vi "BRig_RT_panel_manualTriggering_v0,90.vi"(0 "input_dataMTrig":u16[](array[numeric]), 6 "input_setValues":bool) -> (11 "output_Solenoid_R":bool, 13 "output_Solenoid_L":bool, 14 "output_dataMTrig":u16[](array[numeric]), 15 "output_Audio_L":bool, 16 "output_Audio_R":bool, 17 "output_CueLed":bool, 18 "output_Laser_l1":bool, 19 "output_Laser_l2":bool)   [LabVIEW 2014]
panel:
  in  "warmup_CueSwitch":bool
  out "SolenoidCal_I_R":bool
  out "SolenoidCal_I_L":bool
  in  "CueLed_T":u16=10 caption="Time [ms]"
  in  "Audio_T":u16=10 caption="Time [ms]"
  in  "count_warmup_R_reset":bool
  in  "count_warmup_L_reset":bool
  out "count_warmup_R":u16
  out "count_warmup_L":u16
  in  "warmup_struct":u8(slide) max=2 step=1 scale=0.0..2.0
  in  "warmup":bool caption="WarmUp"
  in  "CueLed":bool
  in  "Laser_Switch":bool
  in  "Laser_T":u16=10 caption="Time [ms]"
  in  "Laser":bool
  in  "Audio_R":bool caption="Trigger Audio"
  in  "Audio_L":bool caption="Trigger Audio"
  in  "RewCalib_R":bool caption="Calibrate_R"
  in  "RewCalib_L":bool caption="Calibrate_L"
  in  "Solenoid_T_R":u16=300 caption="Time [ms]"
  in  "Solenoid_T_L":u16=300 caption="Time [ms]"
  in  "Solenoid_R":bool caption="Solenoid"
  in  "Solenoid_L":bool caption="Solenoid"
  # "WarmUp"
  # "Cue then reward (no lick)\n \nLeft                    Right"
  # "Cue LED\n\nAudio"
  # "Manual Control"
  # "Solenoid\n \nLeft              Right"
  # "Speaker\n \nLeft                    Right"
  # "Laser 1  |  Laser 2"
  # "Cue LED"
  # "Time\n[ms]"
  # "Time\n[ms]"
  # "Power = Min"
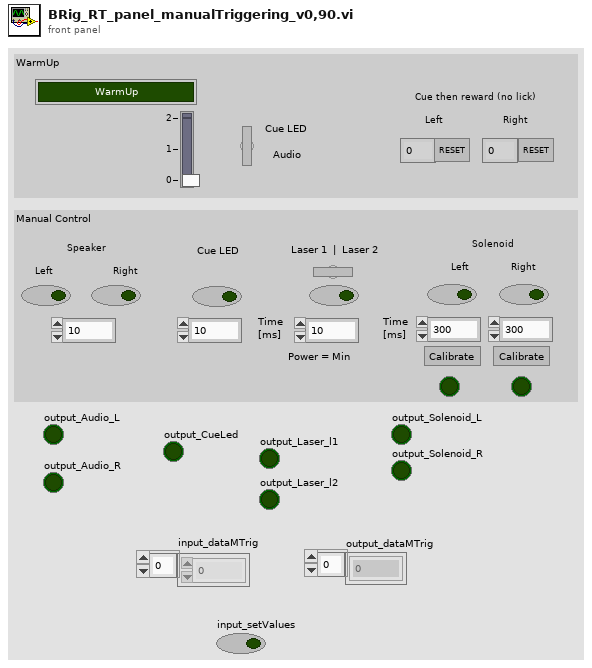
[diagram p1: front panel]
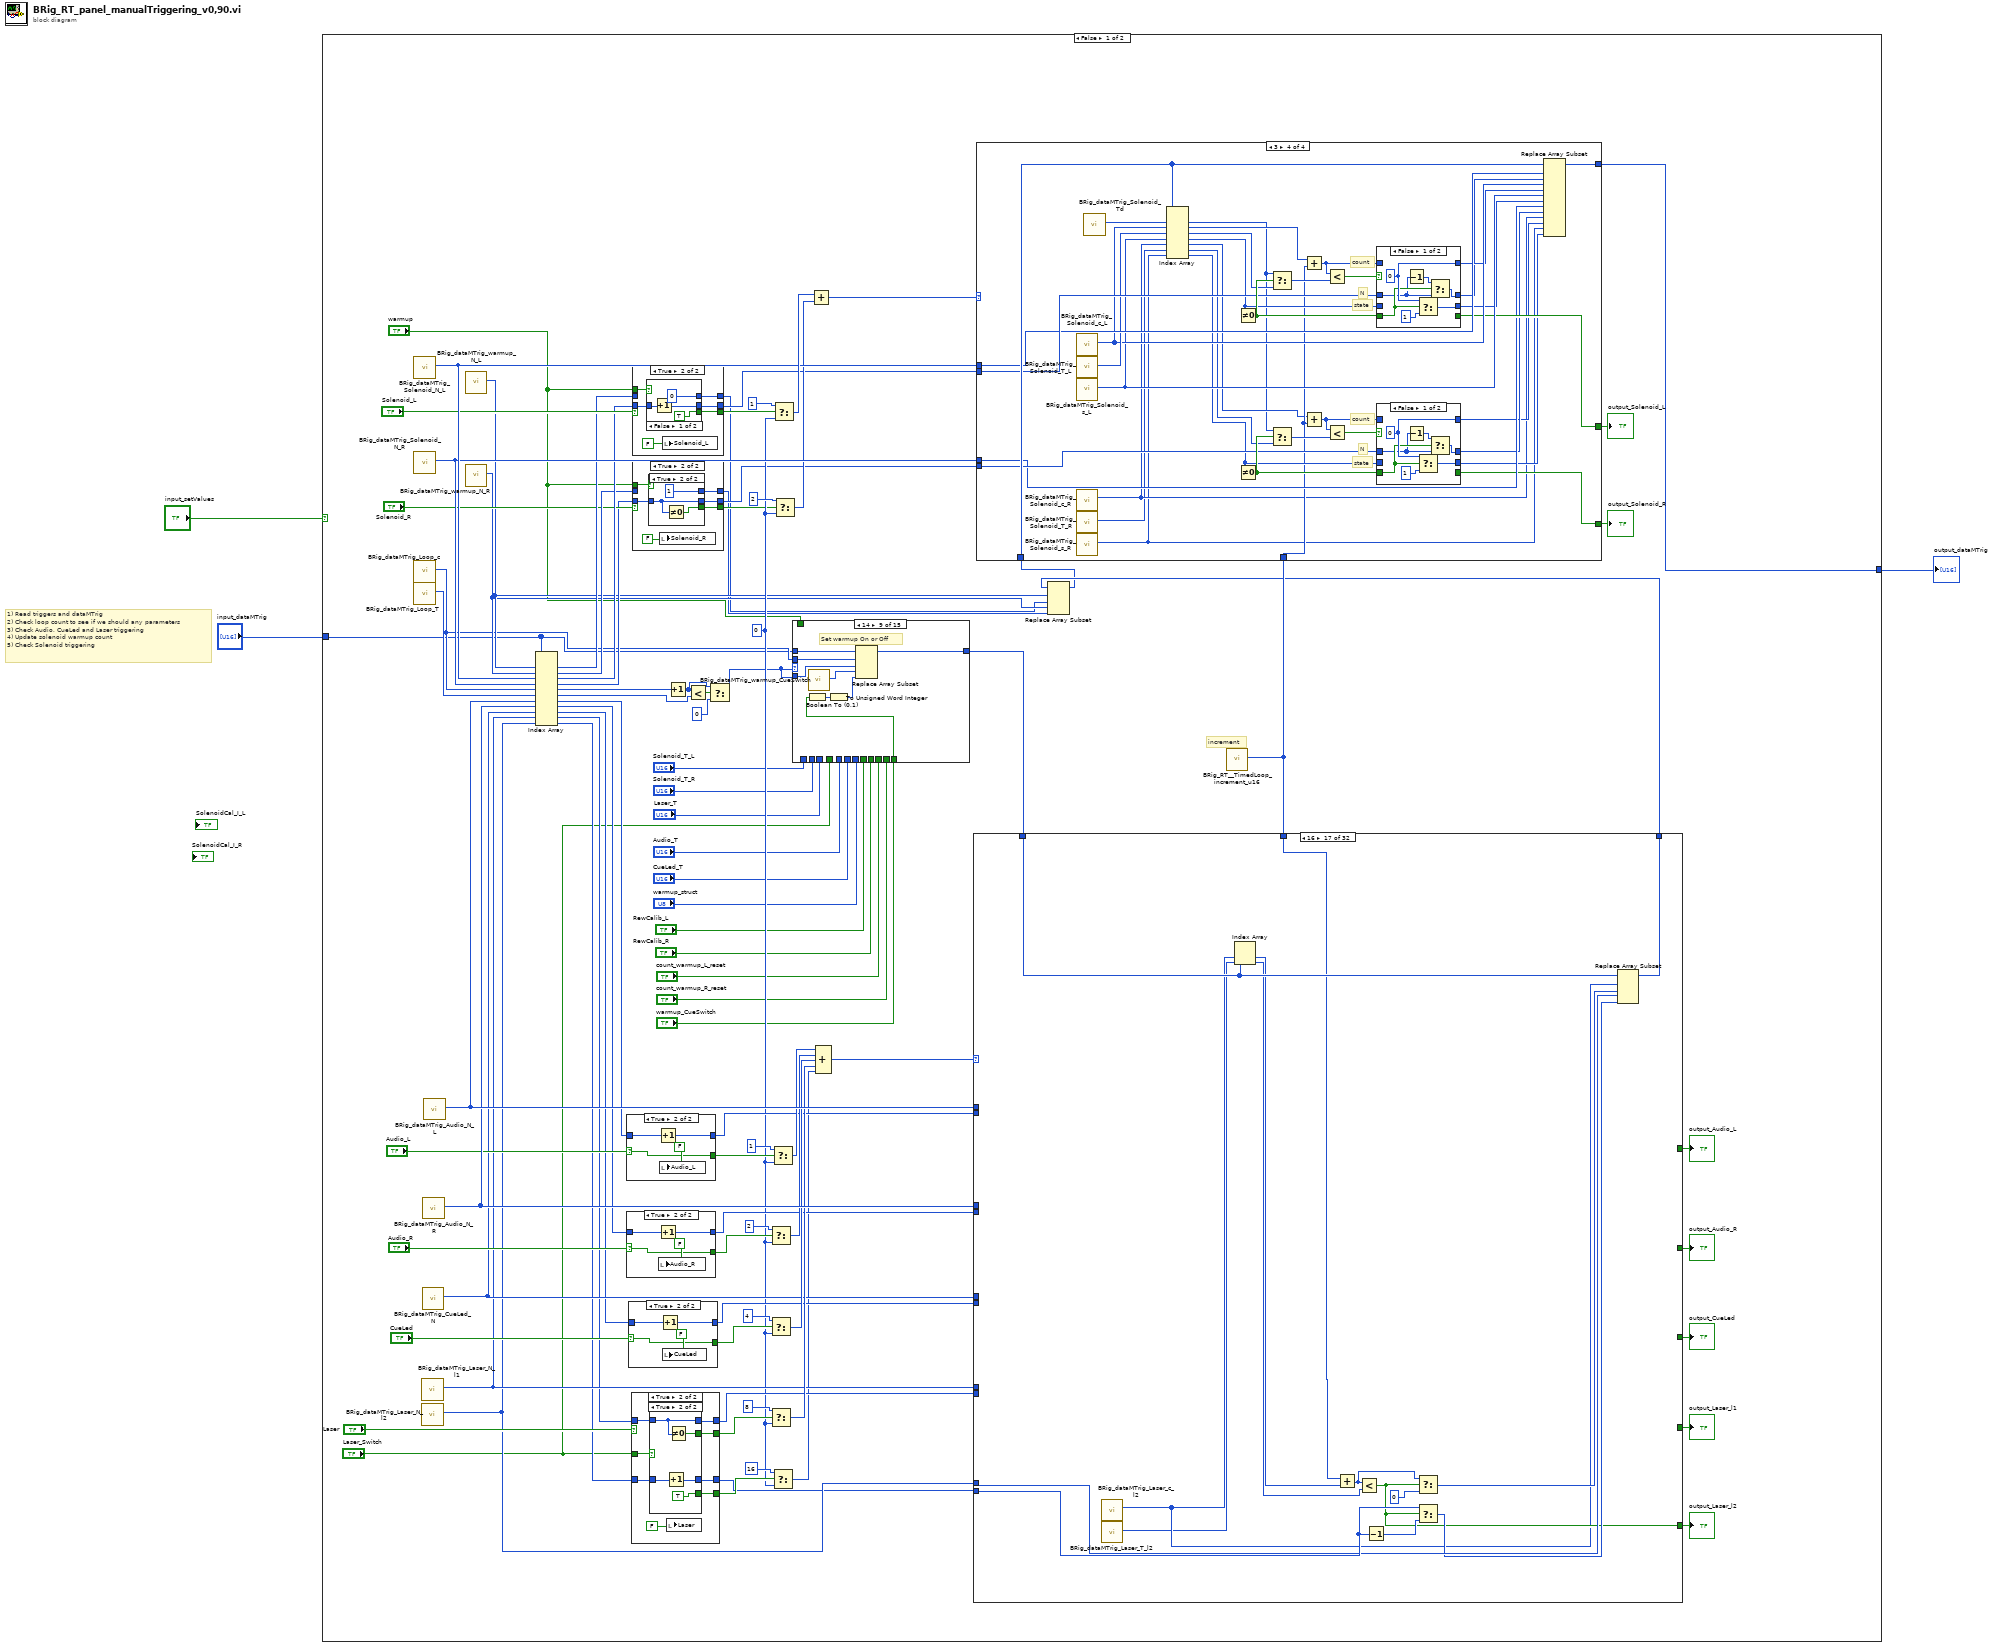
[diagram p0: block diagram]
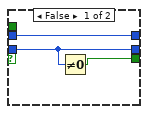
[diagram p2: hidden frame]
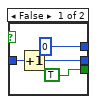
[diagram p3: hidden frame]
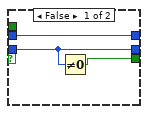
[diagram p4: hidden frame]
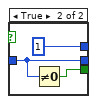
[diagram p5: hidden frame]
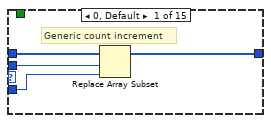
[diagram p6: hidden frame]
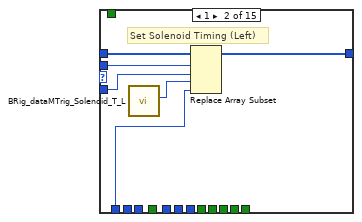
[diagram p7: hidden frame]
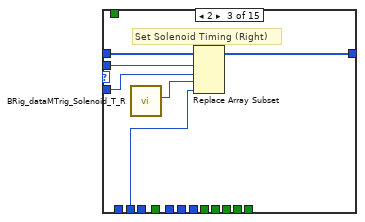
[diagram p8: hidden frame]
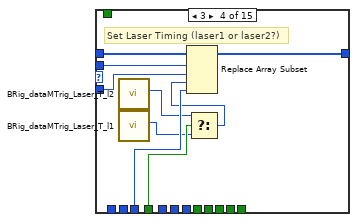
[diagram p9: hidden frame]
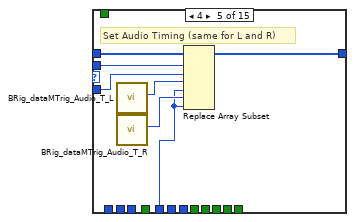
[diagram p10: hidden frame]
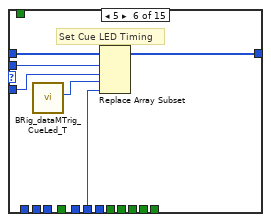
[diagram p11: hidden frame]
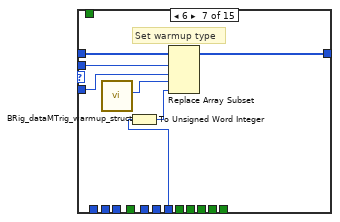
[diagram p12: hidden frame]
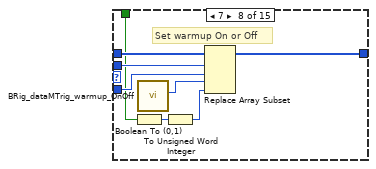
[diagram p13: hidden frame]
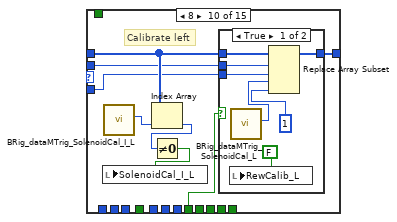
[diagram p14: hidden frame]
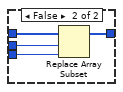
[diagram p15: hidden frame]
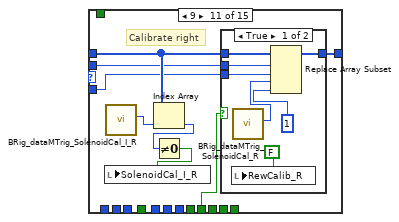
[diagram p16: hidden frame]
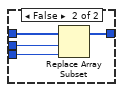
[diagram p17: hidden frame]
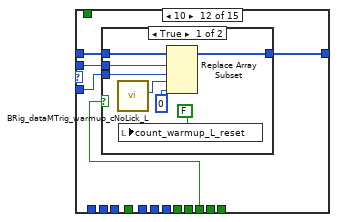
[diagram p18: hidden frame]
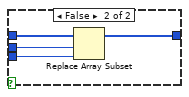
[diagram p19: hidden frame]
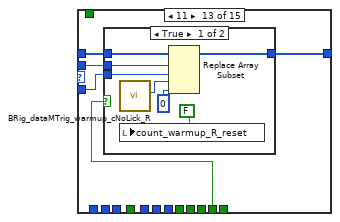
[diagram p20: hidden frame]
diagram:
  # "1) Read triggers and dataMTrig\n2) Check loop count to see if we should any parameters\n3) Check Audio, CueLed and Laser triggering\n4) Update solenoid warmup count\n5) Check Solenoid triggering"
  n1 = case shown="False" "input_setValues" {
    tunnel: [w54 w1492] -> w3
    tunnel: "input_dataMTrig" -> [w7 w1492]
    frame False {
      w39 = u8 0 ("f")
      # "increment"
      n2 = call "BRig_dataMTrig_Solenoid_N_L.vi"() -> ("output_Solenoid_N_L"=w48:i32)  [unwired: 11 in]
      n3 = call "BRig_dataMTrig_Solenoid_N_R.vi"() -> ("output_Solenoid_N_R"=w47:i32)  [unwired: 11 in]
      n4 = call "BRig_dataMTrig_Loop_c.vi"() -> ("output_Loop_c"=w9:i32)  [unwired: 11 in]
      n5 = call "BRig_dataMTrig_Loop_T.vi"() -> ("output_Loop_T"=w52:i32)  [unwired: 11 in]
      n6 = call "BRig_dataMTrig_Laser_N_l1.vi"() -> ("output_Laser_N_l1"=w73:i32)  [unwired: 11 in]
      n7 = call "BRig_dataMTrig_Laser_N_l2.vi"() -> ("output_Laser_N_l2"=w61:i32)  [unwired: 11 in]
      n8 = call "BRig_dataMTrig_CueLed_N.vi"() -> ("output_CueLed_N"=w74:i32)  [unwired: 11 in]
      n9 = call "BRig_dataMTrig_Audio_N_R.vi"() -> ("output_Audio_N_R"=w91:i32)  [unwired: 11 in]
      n10 = call "BRig_dataMTrig_Audio_N_L.vi"() -> ("output_Audio_N_L"=w92:i32)  [unwired: 11 in]
      n11 = call "BRig_dataMTrig_warmup_N_L.vi"() -> ("output_warmup_N_L"=w18:i32)  [unwired: 11 in]
      n12 = call "BRig_dataMTrig_warmup_N_R.vi"() -> ("output_warmup_N_R"=w17:i32)  [unwired: 11 in]
      n13 = Index Array(array=w7, index #1=w18, index #2=w17, index #3=w48, index #4=w47, index #5=w9, index #6=w52, index #7=w92, index #8=w91, index #9=w74, index #10=w73, index #11=w61) -> (element #1=w28:u16, element #2=w25:u16, element #3=w29:u16, element #4=w23:u16, element #5=w42:u16, element #6=w41:u16, element #7=w82:u16, element #8=w78:u16, element #9=w72:u16, element #10=w69:u16, element #11=w65:u16)
      n14 = case shown="True" "Audio_L" {
        selector: "Audio_L" -> [_ w434]
        tunnel: w82 -> [w433 w437]
        tunnel: [w433 w436] -> w81
        tunnel: [w432 w434] -> w80
        frame False {
          n15 = Not Equal To 0?(x=w433) -> (x != 0?=w432:bool)
        }
        frame True {
          n16 = Increment(x=w437) -> (x+1=w436:u16)
          n17 = local write "Audio_L"(FALSE) -> ()
        }
      }
      n18 = case shown="True" "Audio_R" {
        selector: "Audio_R" -> [_ w428]
        tunnel: w78 -> [w427 w431]
        tunnel: [w427 w430] -> w76
        tunnel: [w426 w428] -> w77
        frame False {
          n19 = Not Equal To 0?(x=w427) -> (x != 0?=w426:bool)
        }
        frame True {
          n20 = Increment(x=w431) -> (x+1=w430:u16)
          n21 = local write "Audio_R"(FALSE) -> ()
        }
      }
      n22 = case shown="True" "CueLed" {
        selector: "CueLed" -> [_ w422]
        tunnel: w72 -> [w421 w425]
        tunnel: [w421 w424] -> w71
        tunnel: [w420 w422] -> w70
        frame False {
          n23 = Not Equal To 0?(x=w421) -> (x != 0?=w420:bool)
        }
        frame True {
          n24 = Increment(x=w425) -> (x+1=w424:u16)
          n25 = local write "CueLed"(FALSE) -> ()
        }
      }
      n26 = case shown="True" "Laser" {
        tunnel: w69 -> [w401 w407]
        tunnel: [w401 w406] -> w67
        tunnel: [w400 w405] -> w66
        tunnel: w65 -> [w399 w404]
        tunnel: "Laser_Switch" -> [_ w408]
        tunnel: [w399 w402] -> w60
        tunnel: [w398 w403] -> w63
        frame False {
          n27 = Not Equal To 0?(x=w401) -> (x != 0?=w400:bool)
          n28 = Not Equal To 0?(x=w399) -> (x != 0?=w398:bool)
        }
        frame True {
          n29 = case shown="True" w408 {
            tunnel: w407 -> [w414 w419]
            tunnel: [w413 w419] -> w406
            tunnel: [TRUE w418] -> w405
            tunnel: [w411 w416] -> w402
            tunnel: w404 -> [w411 w417]
            tunnel: [w410 TRUE] -> w403
            frame False {
              n30 = Increment(x=w414) -> (x+1=w413:u16)
              n31 = Not Equal To 0?(x=w411) -> (x != 0?=w410:bool)
            }
            frame True {
              n32 = Increment(x=w417) -> (x+1=w416:u16)
              n33 = Not Equal To 0?(x=w419) -> (x != 0?=w418:bool)
            }
          }
          n34 = local write "Laser"(FALSE) -> ()
        }
      }
      n35 = case shown="True" "Solenoid_L" {
        tunnel: w29 -> [w113 w119]
        tunnel: [w113 w118] -> w26
        tunnel: [w112 w114] -> w27
        tunnel: "warmup" -> [_ w117]
        tunnel: [w111 w116] -> w15
        tunnel: w28 -> [w111 _]
        frame False {
          n36 = Not Equal To 0?(x=w113) -> (x != 0?=w112:bool)
        }
        frame True {
          n37 = case shown="False" w117 {
            tunnel: w119 -> [w123 w125]
            tunnel: [w122 w125] -> w118
            tunnel: [u16 0 u16 1] -> w116
            tunnel: [TRUE w124] -> w114
            frame False {
              n38 = Increment(x=w123) -> (x+1=w122:u16)
            }
            frame True {
              n39 = Not Equal To 0?(x=w125) -> (x != 0?=w124:bool)
            }
          }
          n40 = local write "Solenoid_L"(FALSE) -> ()
        }
      }
      n41 = case shown="True" "Solenoid_R" {
        tunnel: w23 -> [w97 w100]
        tunnel: [w97 w102] -> w21
        tunnel: [w96 w98] -> w22
        tunnel: "warmup" -> [_ w101]
        tunnel: [w95 w99] -> w16
        tunnel: w25 -> [w95 _]
        frame False {
          n42 = Not Equal To 0?(x=w97) -> (x != 0?=w96:bool)
        }
        frame True {
          n43 = case shown="True" w101 {
            tunnel: w100 -> [w107 w109]
            tunnel: [w106 w109] -> w102
            tunnel: [u16 0 u16 1] -> w99
            tunnel: [TRUE w108] -> w98
            frame False {
              n44 = Increment(x=w107) -> (x+1=w106:u16)
            }
            frame True {
              n45 = Not Equal To 0?(x=w109) -> (x != 0?=w108:bool)
            }
          }
          n46 = local write "Solenoid_R"(FALSE) -> ()
        }
      }
      n47 = Increment(x=w42) -> (x+1=w36:u16)
      n48 = Less?(x=w36, y=w41) -> (x < y?=w40:bool)
      n49 = Select(t=w36, s=w40, f=u16 0) -> (s? t:f=w31:u16)
      n50 = Select(t=u8 2, s=w77, f=w39) -> (s? t:f=w88:u8)
      n51 = Select(t=u8 4, s=w70, f=w39) -> (s? t:f=w87:u8)
      n52 = Select(t=u8 8, s=w66, f=w39) -> (s? t:f=w85:u8)
      n53 = Select(t=u8 1, s=w80, f=w39) -> (s? t:f=w89:u8)
      n54 = Select(t=u8 16, s=w63, f=w39) -> (s? t:f=w62:u8)
      n55 = Select(t=u8 1, s=w27, f=w39) -> (s? t:f=w50:u8)
      n56 = Select(t=u8 2, s=w22, f=w39) -> (s? t:f=w45:u8)
      n57 = case shown="14" w31 {
        tunnel: w7 -> [w130 w136 w142 w151 w158 w164 w171 w179 w187 w192 w211 w230 w246 w260 w266]
        tunnel: [w129 w135 w141 w150 w157 w163 w170 w178 w186 w190 w210 w229 w245 w263 w269] -> w37
        tunnel: w31 -> [w127 w133 w139 w148 w155 w161 w168 w176 w184 w188 w208 w227 w243 w261 w267]
        tunnel: w9 -> [w128 w134 w140 w149 w156 w162 w169 w177 w185 w189 w209 w228 w244 w262 w268]
        tunnel: "Solenoid_T_L" -> [_ w131 _ _ _ _ _ _ _ _ _ _ _ _ _]
        tunnel: "Solenoid_T_R" -> [_ _ w137 _ _ _ _ _ _ _ _ _ _ _ _]
        tunnel: "Laser_T" -> [_ _ _ w147 _ _ _ _ _ _ _ _ _ _ _]
        tunnel: "Laser_Switch" -> [_ _ _ w146 _ _ _ _ _ _ _ _ _ _ _]
        tunnel: "Audio_T" -> [_ _ _ _ w152 _ _ _ _ _ _ _ _ _ _]
        tunnel: "CueLed_T" -> [_ _ _ _ _ w159 _ _ _ _ _ _ _ _ _]
        tunnel: "warmup_struct" -> [_ _ _ _ _ _ w166 _ _ _ _ _ _ _ _]
        tunnel: "warmup" -> [_ _ _ _ _ _ _ w172 _ _ _ _ _ _ _]
        tunnel: "RewCalib_L" -> [_ _ _ _ _ _ _ _ _ w191 _ _ _ _ _]
        tunnel: "RewCalib_R" -> [_ _ _ _ _ _ _ _ _ _ w207 _ _ _ _]
        tunnel: "count_warmup_L_reset" -> [_ _ _ _ _ _ _ _ _ _ _ w226 _ _ _]
        tunnel: "count_warmup_R_reset" -> [_ _ _ _ _ _ _ _ _ _ _ _ w242 _ _]
        tunnel: "warmup_CueSwitch" -> [_ _ _ _ _ _ _ _ w181 _ _ _ _ _ _]
        frame 0, Default {
          # "Generic count increment"
          n58 = Replace Array Subset(array=w130, new element=w127, index=w128) -> (w129:u16[])
        }
        frame 1 {
          # "Set Solenoid Timing (Left)"
          n59 = call "BRig_dataMTrig_Solenoid_T_L.vi"() -> ("output_Solenoid_T_L"=w132:i32)  [unwired: 11 in]
          n60 = Replace Array Subset(array=w136, new element #1=w133, index #1=w134, new element #2=w131, index #2=w132) -> (w135:u16[])
        }
        frame 2 {
          # "Set Solenoid Timing (Right)"
          n61 = call "BRig_dataMTrig_Solenoid_T_R.vi"() -> ("output_Solenoid_T_R"=w138:i32)  [unwired: 11 in]
          n62 = Replace Array Subset(array=w142, new element #1=w139, index #1=w140, new element #2=w137, index #2=w138) -> (w141:u16[])
        }
        frame 3 {
          # "Set Laser Timing (laser1 or laser2?)"
          n63 = call "BRig_dataMTrig_Laser_T_l2.vi"() -> ("output_Laser_T_l2"=w144:i32)  [unwired: 11 in]
          n64 = call "BRig_dataMTrig_Laser_T_l1.vi"() -> ("output_Laser_T_l1"=w145:i32)  [unwired: 11 in]
          n65 = Select(t=w144, s=w146, f=w145) -> (s? t:f=w143:i32)
          n66 = Replace Array Subset(array=w151, new element #1=w148, index #1=w149, new element #2=w147, index #2=w143) -> (w150:u16[])
        }
        frame 4 {
          # "Set Audio Timing (same for L and R)"
          n67 = call "BRig_dataMTrig_Audio_T_L.vi"() -> ("output_Audio_T_L"=w154:i32)  [unwired: 11 in]
          n68 = call "BRig_dataMTrig_Audio_T_R.vi"() -> ("output_Audio_T_R"=w153:i32)  [unwired: 11 in]
          n69 = Replace Array Subset(array=w158, new element #1=w155, index #1=w156, new element #2=w152, index #2=w154, new element #3=w152, index #3=w153) -> (w157:u16[])
        }
        frame 5 {
          # "Set Cue LED Timing"
          n70 = call "BRig_dataMTrig_CueLed_T.vi"() -> ("output_CueLed_T"=w160:i32)  [unwired: 11 in]
          n71 = Replace Array Subset(array=w164, new element #1=w161, index #1=w162, new element #2=w159, index #2=w160) -> (w163:u16[])
        }
        frame 6 {
          # "Set warmup type"
          n72 = call "BRig_dataMTrig_warmup_struct.vi"() -> ("output_warmup_struct"=w167:i32)  [unwired: 11 in]
          n73 = To Unsigned Word Integer(number=w166) -> (unsigned 16bit integer=w165:u16)
          n74 = Replace Array Subset(array=w171, new element #1=w168, index #1=w169, new element #2=w165, index #2=w167) -> (w170:u16[])
        }
        frame 7 {
          # "Set warmup On or Off"
          n75 = Boolean To (0,1)(Boolean=w172) -> (0, 1=w173:i16)
          n76 = call "BRig_dataMTrig_warmup_OnOff.vi"() -> ("output_warmup_OnOff"=w174:i32)  [unwired: 11 in]
          n77 = To Unsigned Word Integer(number=w173) -> (unsigned 16bit integer=w175:u16)
          n78 = Replace Array Subset(array=w179, new element #1=w176, index #1=w177, new element #2=w175, index #2=w174) -> (w178:u16[])
        }
        frame 14 {
          # "Set warmup On or Off"
          n79 = Boolean To (0,1)(Boolean=w181) -> (0, 1=w182:i16)
          n80 = call "BRig_dataMTrig_warmup_CueSwitch.vi"() -> ("output_warmup_CueSwitch"=w180:i32)  [unwired: 11 in]
          n81 = To Unsigned Word Integer(number=w182) -> (unsigned 16bit integer=w183:u16)
          n82 = Replace Array Subset(array=w187, new element #1=w184, index #1=w185, new element #2=w183, index #2=w180) -> (w186:u16[])
        }
        frame 8 {
          # "Calibrate left"
          n83 = call "BRig_dataMTrig_SolenoidCal_I_L.vi"() -> ("output_SolenoidCal_I_L"=w195:i32)  [unwired: 11 in]
          n84 = Index Array(array=w192, index=w195) -> (element=w194:u16)
          n85 = Not Equal To 0?(x=w194) -> (x != 0?=w193:bool)
          n86 = local write "SolenoidCal_I_L"(w193) -> ()
          n87 = case shown="True" w191 {
            tunnel: w192 -> [w201 w206]
            tunnel: [w200 w205] -> w190
            tunnel: w189 -> [w199 w204]
            tunnel: w188 -> [w198 w203]
            frame True {
              n88 = local write "RewCalib_L"(FALSE) -> ()
              n89 = call "BRig_dataMTrig_SolenoidCal_L.vi"() -> ("output_SolenoidCal_L"=w197:i32)  [unwired: 11 in]
              n90 = Replace Array Subset(array=w201, new element #1=w198, index #1=w199, new element #2=u16 1 ("new element/subarray"), index #2=w197) -> (w200:u16[])
            }
            frame False {
              n91 = Replace Array Subset(array=w206, new element=w203, index=w204) -> (w205:u16[])
            }
          }
        }
        frame 9 {
          # "Calibrate right"
          n92 = call "BRig_dataMTrig_SolenoidCal_I_R.vi"() -> ("output_SolenoidCal_I_R"=w214:i32)  [unwired: 11 in]
          n93 = Index Array(array=w211, index=w214) -> (element=w213:u16)
          n94 = Not Equal To 0?(x=w213) -> (x != 0?=w212:bool)
          n95 = local write "SolenoidCal_I_R"(w212) -> ()
          n96 = case shown="True" w207 {
            tunnel: w211 -> [w220 w225]
            tunnel: [w219 w224] -> w210
            tunnel: w209 -> [w218 w223]
            tunnel: w208 -> [w217 w222]
            frame True {
              n97 = local write "RewCalib_R"(FALSE) -> ()
              n98 = call "BRig_dataMTrig_SolenoidCal_R.vi"() -> ("output_SolenoidCal_R"=w216:i32)  [unwired: 11 in]
              n99 = Replace Array Subset(array=w220, new element #1=w217, index #1=w218, new element #2=u16 1 ("new element/subarray"), index #2=w216) -> (w219:u16[])
            }
            frame False {
              n100 = Replace Array Subset(array=w225, new element=w222, index=w223) -> (w224:u16[])
            }
          }
        }
        frame 10 {
          n101 = case shown="True" w226 {
            tunnel: w230 -> [w237 w241]
            tunnel: [w236 w240] -> w229
            tunnel: w228 -> [w235 w239]
            tunnel: w227 -> [w234 w238]
            frame True {
              n102 = call "BRig_dataMTrig_warmup_cNoLick_L.vi"() -> ("output_warmup_cNoLick_L"=w233:i32)  [unwired: 11 in]
              n103 = local write "count_warmup_L_reset"(FALSE ("count_warmup_L_reset")) -> ()
              n104 = Replace Array Subset(array=w237, new element #1=w234, index #1=w235, new element #2=u16 0 ("new element/subarray"), index #2=w233) -> (w236:u16[])
            }
            frame False {
              n105 = Replace Array Subset(array=w241, new element=w238, index=w239) -> (w240:u16[])
            }
          }
        }
        frame 11 {
          n106 = case shown="True" w242 {
            tunnel: w246 -> [w253 w257]
            tunnel: [w252 w256] -> w245
            tunnel: w244 -> [w251 w255]
            tunnel: w243 -> [w250 w254]
            frame True {
              n107 = call "BRig_dataMTrig_warmup_cNoLick_R.vi"() -> ("output_warmup_cNoLick_R"=w247:i32)  [unwired: 11 in]
              n108 = local write "count_warmup_R_reset"(FALSE ("count_warmup_L_reset")) -> ()
              n109 = Replace Array Subset(array=w253, new element #1=w250, index #1=w251, new element #2=u16 0 ("new element/subarray"), index #2=w247) -> (w252:u16[])
            }
            frame False {
              n110 = Replace Array Subset(array=w257, new element=w254, index=w255) -> (w256:u16[])
            }
          }
        }
        frame 12 {
          n111 = call "BRig_dataMTrig_warmup_cNoLick_L.vi"() -> ("output_warmup_cNoLick_L"=w259:i32)  [unwired: 11 in]
          n112 = Replace Array Subset(array=w260, new element=w261, index=w262) -> (w263:u16[])
          n113 = Index Array(array=w260, index=w259) -> (element=→"count_warmup_L":u16)
        }
        frame 13 {
          n114 = call "BRig_dataMTrig_warmup_cNoLick_R.vi"() -> ("output_warmup_cNoLick_R"=w265:i32)  [unwired: 11 in]
          n115 = Replace Array Subset(array=w266, new element=w267, index=w268) -> (w269:u16[])
          n116 = Index Array(array=w266, index=w265) -> (element=→"count_warmup_R":u16)
        }
      }
      n117 = Add(x=w50, y=w45) -> (x+y=w49:u8)
      n118 = Compound Arithmetic op=ADD(w89, w88, w87, w85, w62) -> (w84:u8)
      n119 = call "BRig_RT__TimedLoop_increment_u16.vi"() -> ("output_increment__u16"=w53:u16)  [unwired: 11 in]
      n120 = case shown="16" w84 {
        tunnel: w37 -> [w438 w443 w458 w476 w502 w524 w547 w577 w618 w636 w669 w693 w731 w767 w800 w842 w882 w900 w927 w957 w995 w1029 w1064 w1106 w1158 w1194 w1233 w1281 w1319 w1367 w1412 w1466]
        tunnel: w53 -> [_ w444 w459 w477 w503 w525 w548 w578 w606 w626 w655 w680 w716 w750 w782 w821 w874 w891 w918 w945 w984 w1018 w1050 w1089 w1138 w1172 w1211 w1257 w1294 w1340 w1384 w1435]
        tunnel: [w438 w442 w457 w475 w501 w523 w546 w576 w617 w635 w668 w692 w730 w766 w799 w841 w881 w899 w926 w956 w994 w1028 w1063 w1105 w1157 w1193 w1232 w1280 w1318 w1366 w1411 w1465] -> w20
        tunnel: w92 -> [_ w440 _ w472 _ w520 _ w572 _ w633 _ w689 _ w744 _ w837 _ w897 _ w953 _ w1025 _ w1101 _ w1162 _ w1241 _ w1331 _ w1461]
        tunnel: w81 -> [_ w439 _ w471 _ w519 _ w571 _ w632 _ w688 _ w763 _ w836 _ w896 _ w952 _ w1024 _ w1100 _ w1191 _ w1277 _ w1363 _ w1460]
        tunnel: [_ w441 _ w474 _ w522 _ w575 _ w634 _ w691 _ w765 _ w840 _ w898 _ w955 _ w1027 _ w1104 _ w1192 _ w1279 _ w1365 _ w1464] -> w59
        tunnel: [_ _ w456 w473 _ _ w545 w574 _ _ w667 w690 _ _ w798 w839 _ _ w925 w954 _ _ w1062 w1103 _ _ w1231 w1278 _ _ w1410 w1463] -> w58
        tunnel: [_ _ _ _ w500 w521 w544 w573 _ _ _ _ w729 w764 w797 w838 _ _ _ _ w993 w1026 w1061 w1102 _ _ _ _ w1317 w1364 w1409 w1462] -> w57
        tunnel: w91 -> [_ _ w455 w470 _ _ w543 w570 _ _ w649 w687 _ _ w796 w835 _ _ w924 w951 _ _ w1060 w1099 _ _ w1202 w1245 _ _ w1408 w1459]
        tunnel: w76 -> [_ _ w454 w469 _ _ w542 w569 _ _ w666 w686 _ _ w795 w834 _ _ w923 w950 _ _ w1059 w1098 _ _ w1230 w1276 _ _ w1407 w1458]
        tunnel: w74 -> [_ _ _ _ w499 w514 w541 w568 _ _ _ _ w728 w762 w794 w833 _ _ _ _ w992 w1015 w1058 w1097 _ _ _ _ w1316 w1362 w1406 w1457]
        tunnel: w71 -> [_ _ _ _ w498 w518 w540 w567 _ _ _ _ w727 w761 w793 w832 _ _ _ _ w991 w1023 w1057 w1096 _ _ _ _ w1315 w1361 w1405 w1456]
        tunnel: w73 -> [_ _ _ _ _ _ _ _ w611 w622 w660 w676 w721 w755 w787 w826 _ _ _ _ _ _ _ _ w1151 w1185 w1224 w1270 w1309 w1355 w1399 w1450]
        tunnel: w67 -> [_ _ _ _ _ _ _ _ w613 w628 w662 w682 w723 w757 w789 w828 _ _ _ _ _ _ _ _ w1153 w1187 w1226 w1272 w1311 w1357 w1401 w1452]
        tunnel: [_ _ _ _ _ _ _ _ w612 w627 w661 w681 w722 w756 w788 w827 _ _ _ _ _ _ _ _ w1152 w1186 w1225 w1271 w1310 w1356 w1400 w1451] -> w56
        tunnel: w61 -> [_ _ _ _ _ _ _ _ _ _ _ _ _ _ _ _ w872 w888 w915 w940 w979 w1012 w1047 w1086 w1136 w1170 w1209 w1255 w1292 w1338 w1382 w1433]
        tunnel: w60 -> [_ _ _ _ _ _ _ _ _ _ _ _ _ _ _ _ w877 w892 w919 w946 w985 w1019 w1051 w1090 w1141 w1175 w1214 w1260 w1297 w1343 w1387 w1438]
        tunnel: [_ _ _ _ _ _ _ _ _ _ _ _ _ _ _ _ w870 w890 w917 w944 w983 w1017 w1049 w1088 w1134 w1168 w1207 w1253 w1290 w1336 w1380 w1431] -> w55
        frame 0, Default {
        }
        frame 1 {
          # "Audio_L"
          # "Tcycle"
          # "count"
          n121 = call "BRig_dataMTrig_Audio_c_L.vi"() -> ("output_Audio_c_L"=w445:i32)  [unwired: 11 in]
          n122 = call "BRig_dataMTrig_Audio_T_L.vi"() -> ("output_Audio_T_L"=w450:i32)  [unwired: 11 in]
          n123 = Index Array(array=w443, index #1=w445, index #2=w450) -> (element #1=w449:u16, element #2=w448:u16)
          n124 = Add(x=w444, y=w449) -> (x+y=w452:u16)
          n125 = Less?(x=w452, y=w448) -> (x < y?=w441:bool)
          n126 = Decrement(x=w439) -> (x-1=w453:u16)
          n127 = Select(t=w452, s=w441, f=u16 0) -> (s? t:f=w447:u16)
          n128 = Select(t=w439, s=w441, f=w453) -> (s? t:f=w446:u16)
          n129 = Replace Array Subset(array=w443, new element #1=w447, index #1=w445, new element #2=w446, index #2=w440) -> (w442:u16[])
        }
        frame 2 {
          # "Audio_R"
          # "Tcycle"
          # "count"
          n130 = call "BRig_dataMTrig_Audio_c_R.vi"() -> ("output_Audio_c_R"=w462:i32)  [unwired: 11 in]
          n131 = call "BRig_dataMTrig_Audio_T_R.vi"() -> ("output_Audio_T_R"=w463:i32)  [unwired: 11 in]
          n132 = Index Array(array=w458, index #1=w462, index #2=w463) -> (element #1=w465:u16, element #2=w464:u16)
          n133 = Add(x=w459, y=w465) -> (x+y=w467:u16)
          n134 = Less?(x=w467, y=w464) -> (x < y?=w456:bool)
          n135 = Decrement(x=w454) -> (x-1=w468:u16)
          n136 = Select(t=w467, s=w456, f=u16 0) -> (s? t:f=w461:u16)
          n137 = Select(t=w454, s=w456, f=w468) -> (s? t:f=w460:u16)
          n138 = Replace Array Subset(array=w458, new element #1=w461, index #1=w462, new element #2=w460, index #2=w455) -> (w457:u16[])
        }
        frame 3 {
          # "Audio_R"
          # "Tcycle"
          # "count"
          # "Audio_L"
          # "Tcycle"
          # "count"
          n139 = call "BRig_dataMTrig_Audio_c_L.vi"() -> ("output_Audio_c_L"=w487:i32)  [unwired: 11 in]
          n140 = call "BRig_dataMTrig_Audio_T_L.vi"() -> ("output_Audio_T_L"=w492:i32)  [unwired: 11 in]
          n141 = call "BRig_dataMTrig_Audio_c_R.vi"() -> ("output_Audio_c_R"=w480:i32)  [unwired: 11 in]
          n142 = call "BRig_dataMTrig_Audio_T_R.vi"() -> ("output_Audio_T_R"=w481:i32)  [unwired: 11 in]
          n143 = Index Array(array=w476, index #1=w487, index #2=w492, index #3=w480, index #4=w481) -> (element #1=w491:u16, element #2=w490:u16, element #3=w483:u16, element #4=w482:u16)
          n144 = Add(x=w477, y=w491) -> (x+y=w494:u16)
          n145 = Add(x=w477, y=w483) -> (x+y=w485:u16)
          n146 = Less?(x=w494, y=w490) -> (x < y?=w474:bool)
          n147 = Less?(x=w485, y=w482) -> (x < y?=w473:bool)
          n148 = Decrement(x=w471) -> (x-1=w495:u16)
          n149 = Decrement(x=w469) -> (x-1=w486:u16)
          n150 = Select(t=w494, s=w474, f=u16 0) -> (s? t:f=w489:u16)
          n151 = Select(t=w471, s=w474, f=w495) -> (s? t:f=w488:u16)
          n152 = Select(t=w485, s=w473, f=u16 0) -> (s? t:f=w479:u16)
          n153 = Select(t=w469, s=w473, f=w486) -> (s? t:f=w478:u16)
          n154 = Replace Array Subset(array=w476, new element #1=w489, index #1=w487, new element #2=w488, index #2=w472, new element #3=w479, index #3=w480, new element #4=w478, index #4=w470) -> (w475:u16[])
        }
        frame 4 {
          n155 = call "BRig_dataMTrig_CueLed_c.vi"() -> ("output_CueLed_c"=w497:i32)  [unwired: 11 in]
          n156 = call "BRig_dataMTrig_CueLed_T.vi"() -> ("output_CueLed_T"=w496:i32)  [unwired: 11 in]
          n157 = Index Array(array=w502, index #1=w497, index #2=w496) -> (element #1=w507:u16, element #2=w506:u16)
          n158 = Add(x=w503, y=w507) -> (x+y=w509:u16)
          n159 = Less?(x=w509, y=w506) -> (x < y?=w500:bool)
          n160 = Decrement(x=w498) -> (x-1=w510:u16)
          n161 = Select(t=w509, s=w500, f=u16 0) -> (s? t:f=w505:u16)
          n162 = Select(t=w498, s=w500, f=w510) -> (s? t:f=w504:u16)
          n163 = Replace Array Subset(array=w502, new element #1=w505, index #1=w497, new element #2=w504, index #2=w499) -> (w501:u16[])
        }
        frame 5 {
          # "Audio_L"
          # "Tcycle"
          # "count"
          n164 = call "BRig_dataMTrig_CueLed_c.vi"() -> ("output_CueLed_c"=w512:i32)  [unwired: 11 in]
          n165 = call "BRig_dataMTrig_CueLed_T.vi"() -> ("output_CueLed_T"=w511:i32)  [unwired: 11 in]
          n166 = call "BRig_dataMTrig_Audio_c_L.vi"() -> ("output_Audio_c_L"=w529:i32)  [unwired: 11 in]
          n167 = call "BRig_dataMTrig_Audio_T_L.vi"() -> ("output_Audio_T_L"=w534:i32)  [unwired: 11 in]
          n168 = Index Array(array=w524, index #1=w529, index #2=w534, index #3=w512, index #4=w511) -> (element #1=w533:u16, element #2=w532:u16, element #3=w517:u16, element #4=w516:u16)
          n169 = Add(x=w525, y=w533) -> (x+y=w536:u16)
          n170 = Add(x=w525, y=w517) -> (x+y=w527:u16)
          n171 = Less?(x=w536, y=w532) -> (x < y?=w522:bool)
          n172 = Less?(x=w527, y=w516) -> (x < y?=w521:bool)
          n173 = Decrement(x=w519) -> (x-1=w537:u16)
          n174 = Decrement(x=w518) -> (x-1=w528:u16)
          n175 = Select(t=w536, s=w522, f=u16 0) -> (s? t:f=w531:u16)
          n176 = Select(t=w519, s=w522, f=w537) -> (s? t:f=w530:u16)
          n177 = Select(t=w527, s=w521, f=u16 0) -> (s? t:f=w515:u16)
          n178 = Select(t=w518, s=w521, f=w528) -> (s? t:f=w513:u16)
          n179 = Replace Array Subset(array=w524, new element #1=w531, index #1=w529, new element #2=w530, index #2=w520, new element #3=w515, index #3=w512, new element #4=w513, index #4=w514) -> (w523:u16[])
        }
        frame 6 {
          # "Audio_R"
          # "Tcycle"
          # "count"
          n180 = call "BRig_dataMTrig_CueLed_c.vi"() -> ("output_CueLed_c"=w539:i32)  [unwired: 11 in]
          n181 = call "BRig_dataMTrig_CueLed_T.vi"() -> ("output_CueLed_T"=w538:i32)  [unwired: 11 in]
          n182 = call "BRig_dataMTrig_Audio_c_R.vi"() -> ("output_Audio_c_R"=w558:i32)  [unwired: 11 in]
          n183 = call "BRig_dataMTrig_Audio_T_R.vi"() -> ("output_Audio_T_R"=w559:i32)  [unwired: 11 in]
          n184 = Index Array(array=w547, index #1=w558, index #2=w559, index #3=w539, index #4=w538) -> (element #1=w561:u16, element #2=w560:u16, element #3=w552:u16, element #4=w551:u16)
          n185 = Add(x=w548, y=w561) -> (x+y=w563:u16)
          n186 = Add(x=w548, y=w552) -> (x+y=w554:u16)
          n187 = Less?(x=w563, y=w560) -> (x < y?=w545:bool)
          n188 = Less?(x=w554, y=w551) -> (x < y?=w544:bool)
          n189 = Decrement(x=w542) -> (x-1=w564:u16)
          n190 = Decrement(x=w540) -> (x-1=w555:u16)
          n191 = Select(t=w563, s=w545, f=u16 0) -> (s? t:f=w557:u16)
          n192 = Select(t=w542, s=w545, f=w564) -> (s? t:f=w556:u16)
          n193 = Select(t=w554, s=w544, f=u16 0) -> (s? t:f=w550:u16)
          n194 = Select(t=w540, s=w544, f=w555) -> (s? t:f=w549:u16)
          n195 = Replace Array Subset(array=w547, new element #1=w557, index #1=w558, new element #2=w556, index #2=w543, new element #3=w550, index #3=w539, new element #4=w549, index #4=w541) -> (w546:u16[])
        }
        frame 7 {
          # "Audio_R"
          # "Tcycle"
          # "count"
          # "Audio_L"
          # "Tcycle"
          # "count"
          n196 = call "BRig_dataMTrig_CueLed_c.vi"() -> ("output_CueLed_c"=w566:i32)  [unwired: 11 in]
          n197 = call "BRig_dataMTrig_CueLed_T.vi"() -> ("output_CueLed_T"=w565:i32)  [unwired: 11 in]
          n198 = call "BRig_dataMTrig_Audio_c_L.vi"() -> ("output_Audio_c_L"=w595:i32)  [unwired: 11 in]
          n199 = call "BRig_dataMTrig_Audio_T_L.vi"() -> ("output_Audio_T_L"=w600:i32)  [unwired: 11 in]
          n200 = call "BRig_dataMTrig_Audio_c_R.vi"() -> ("output_Audio_c_R"=w588:i32)  [unwired: 11 in]
          n201 = call "BRig_dataMTrig_Audio_T_R.vi"() -> ("output_Audio_T_R"=w589:i32)  [unwired: 11 in]
          n202 = Index Array(array=w577, index #1=w595, index #2=w600, index #3=w588, index #4=w589, index #5=w566, index #6=w565) -> (element #1=w599:u16, element #2=w598:u16, element #3=w591:u16, element #4=w590:u16, element #5=w582:u16, element #6=w581:u16)
          n203 = Add(x=w578, y=w599) -> (x+y=w602:u16)
          n204 = Add(x=w578, y=w591) -> (x+y=w593:u16)
          n205 = Add(x=w578, y=w582) -> (x+y=w584:u16)
          n206 = Less?(x=w602, y=w598) -> (x < y?=w575:bool)
          n207 = Less?(x=w593, y=w590) -> (x < y?=w574:bool)
          n208 = Less?(x=w584, y=w581) -> (x < y?=w573:bool)
          n209 = Decrement(x=w571) -> (x-1=w603:u16)
          n210 = Decrement(x=w569) -> (x-1=w594:u16)
          n211 = Decrement(x=w567) -> (x-1=w585:u16)
          n212 = Select(t=w602, s=w575, f=u16 0) -> (s? t:f=w597:u16)
          n213 = Select(t=w571, s=w575, f=w603) -> (s? t:f=w596:u16)
          n214 = Select(t=w593, s=w574, f=u16 0) -> (s? t:f=w587:u16)
          n215 = Select(t=w569, s=w574, f=w594) -> (s? t:f=w586:u16)
          n216 = Select(t=w584, s=w573, f=u16 0) -> (s? t:f=w580:u16)
          n217 = Select(t=w567, s=w573, f=w585) -> (s? t:f=w579:u16)
          n218 = Replace Array Subset(array=w577, new element #1=w597, index #1=w595, new element #2=w596, index #2=w572, new element #3=w587, index #3=w588, new element #4=w586, index #4=w570, new element #5=w580, index #5=w566, new element #6=w579, index #6=w568) -> (w576:u16[])
        }
        frame 8 {
          n219 = call "BRig_dataMTrig_Laser_c_l1.vi"() -> ("output_Laser_c_l1"=w605:i32)  [unwired: 11 in]
          n220 = call "BRig_dataMTrig_Laser_T_l1.vi"() -> ("output_Laser_T_l1"=w604:i32)  [unwired: 11 in]
          n221 = Index Array(array=w618, index #1=w605, index #2=w604) -> (element #1=w608:u16, element #2=w607:u16)
          n222 = Add(x=w606, y=w608) -> (x+y=w615:u16)
          n223 = Less?(x=w615, y=w607) -> (x < y?=w612:bool)
          n224 = Decrement(x=w613) -> (x-1=w616:u16)
          n225 = Select(t=w615, s=w612, f=u16 0) -> (s? t:f=w610:u16)
          n226 = Select(t=w613, s=w612, f=w616) -> (s? t:f=w609:u16)
          n227 = Replace Array Subset(array=w618, new element #1=w610, index #1=w605, new element #2=w609, index #2=w611) -> (w617:u16[])
        }
        frame 9 {
          # "Audio_L"
          # "Tcycle"
          # "count"
          n228 = call "BRig_dataMTrig_Laser_c_l1.vi"() -> ("output_Laser_c_l1"=w620:i32)  [unwired: 11 in]
          n229 = call "BRig_dataMTrig_Laser_T_l1.vi"() -> ("output_Laser_T_l1"=w619:i32)  [unwired: 11 in]
          n230 = call "BRig_dataMTrig_Audio_c_L.vi"() -> ("output_Audio_c_L"=w637:i32)  [unwired: 11 in]
          n231 = call "BRig_dataMTrig_Audio_T_L.vi"() -> ("output_Audio_T_L"=w642:i32)  [unwired: 11 in]
          n232 = Index Array(array=w636, index #1=w637, index #2=w642, index #3=w620, index #4=w619) -> (element #1=w641:u16, element #2=w640:u16, element #3=w625:u16, element #4=w624:u16)
          n233 = Add(x=w626, y=w641) -> (x+y=w644:u16)
          n234 = Add(x=w626, y=w625) -> (x+y=w630:u16)
          n235 = Less?(x=w644, y=w640) -> (x < y?=w634:bool)
          n236 = Less?(x=w630, y=w624) -> (x < y?=w627:bool)
          n237 = Decrement(x=w632) -> (x-1=w645:u16)
          n238 = Decrement(x=w628) -> (x-1=w631:u16)
          n239 = Select(t=w644, s=w634, f=u16 0) -> (s? t:f=w639:u16)
          n240 = Select(t=w632, s=w634, f=w645) -> (s? t:f=w638:u16)
          n241 = Select(t=w630, s=w627, f=u16 0) -> (s? t:f=w623:u16)
          n242 = Select(t=w628, s=w627, f=w631) -> (s? t:f=w621:u16)
          n243 = Replace Array Subset(array=w636, new element #1=w639, index #1=w637, new element #2=w638, index #2=w633, new element #3=w623, index #3=w620, new element #4=w621, index #4=w622) -> (w635:u16[])
        }
        frame 10 {
          # "Audio_R"
          # "Tcycle"
          # "count"
          n244 = call "BRig_dataMTrig_Laser_c_l1.vi"() -> ("output_Laser_c_l1"=w647:i32)  [unwired: 11 in]
          n245 = call "BRig_dataMTrig_Laser_T_l1.vi"() -> ("output_Laser_T_l1"=w646:i32)  [unwired: 11 in]
          n246 = call "BRig_dataMTrig_Audio_c_R.vi"() -> ("output_Audio_c_R"=w651:i32)  [unwired: 11 in]
          n247 = call "BRig_dataMTrig_Audio_T_R.vi"() -> ("output_Audio_T_R"=w654:i32)  [unwired: 11 in]
          n248 = Index Array(array=w669, index #1=w651, index #2=w654, index #3=w647, index #4=w646) -> (element #1=w653:u16, element #2=w652:u16, element #3=w657:u16, element #4=w656:u16)
          n249 = Add(x=w655, y=w653) -> (x+y=w671:u16)
          n250 = Add(x=w655, y=w657) -> (x+y=w664:u16)
          n251 = Less?(x=w671, y=w652) -> (x < y?=w667:bool)
          n252 = Less?(x=w664, y=w656) -> (x < y?=w661:bool)
          n253 = Decrement(x=w666) -> (x-1=w672:u16)
          n254 = Decrement(x=w662) -> (x-1=w665:u16)
          n255 = Select(t=w671, s=w667, f=u16 0) -> (s? t:f=w650:u16)
          n256 = Select(t=w666, s=w667, f=w672) -> (s? t:f=w648:u16)
          n257 = Select(t=w664, s=w661, f=u16 0) -> (s? t:f=w659:u16)
          n258 = Select(t=w662, s=w661, f=w665) -> (s? t:f=w658:u16)
          n259 = Replace Array Subset(array=w669, new element #1=w650, index #1=w651, new element #2=w648, index #2=w649, new element #3=w659, index #3=w647, new element #4=w658, index #4=w660) -> (w668:u16[])
        }
        frame 11 {
          # "Audio_R"
          # "Tcycle"
          # "count"
          # "Audio_L"
          # "Tcycle"
          # "count"
          n260 = call "BRig_dataMTrig_Laser_c_l1.vi"() -> ("output_Laser_c_l1"=w674:i32)  [unwired: 11 in]
          n261 = call "BRig_dataMTrig_Laser_T_l1.vi"() -> ("output_Laser_T_l1"=w673:i32)  [unwired: 11 in]
          n262 = call "BRig_dataMTrig_Audio_c_L.vi"() -> ("output_Audio_c_L"=w703:i32)  [unwired: 11 in]
          n263 = call "BRig_dataMTrig_Audio_T_L.vi"() -> ("output_Audio_T_L"=w708:i32)  [unwired: 11 in]
          n264 = call "BRig_dataMTrig_Audio_c_R.vi"() -> ("output_Audio_c_R"=w696:i32)  [unwired: 11 in]
          n265 = call "BRig_dataMTrig_Audio_T_R.vi"() -> ("output_Audio_T_R"=w697:i32)  [unwired: 11 in]
          n266 = Index Array(array=w693, index #1=w703, index #2=w708, index #3=w696, index #4=w697, index #5=w674, index #6=w673) -> (element #1=w707:u16, element #2=w706:u16, element #3=w699:u16, element #4=w698:u16, element #5=w679:u16, element #6=w678:u16)
          n267 = Add(x=w680, y=w707) -> (x+y=w710:u16)
          n268 = Add(x=w680, y=w699) -> (x+y=w701:u16)
          n269 = Add(x=w680, y=w679) -> (x+y=w684:u16)
          n270 = Less?(x=w710, y=w706) -> (x < y?=w691:bool)
          n271 = Less?(x=w701, y=w698) -> (x < y?=w690:bool)
          n272 = Less?(x=w684, y=w678) -> (x < y?=w681:bool)
          n273 = Decrement(x=w688) -> (x-1=w711:u16)
          n274 = Decrement(x=w686) -> (x-1=w702:u16)
          n275 = Decrement(x=w682) -> (x-1=w685:u16)
          n276 = Select(t=w710, s=w691, f=u16 0) -> (s? t:f=w705:u16)
          n277 = Select(t=w688, s=w691, f=w711) -> (s? t:f=w704:u16)
          n278 = Select(t=w701, s=w690, f=u16 0) -> (s? t:f=w695:u16)
          n279 = Select(t=w686, s=w690, f=w702) -> (s? t:f=w694:u16)
          n280 = Select(t=w684, s=w681, f=u16 0) -> (s? t:f=w677:u16)
          n281 = Select(t=w682, s=w681, f=w685) -> (s? t:f=w675:u16)
          n282 = Replace Array Subset(array=w693, new element #1=w705, index #1=w703, new element #2=w704, index #2=w689, new element #3=w695, index #3=w696, new element #4=w694, index #4=w687, new element #5=w677, index #5=w674, new element #6=w675, index #6=w676) -> (w692:u16[])
        }
        frame 12 {
          n283 = call "BRig_dataMTrig_CueLed_c.vi"() -> ("output_CueLed_c"=w713:i32)  [unwired: 11 in]
          n284 = call "BRig_dataMTrig_CueLed_T.vi"() -> ("output_CueLed_T"=w712:i32)  [unwired: 11 in]
          n285 = call "BRig_dataMTrig_Laser_c_l1.vi"() -> ("output_Laser_c_l1"=w715:i32)  [unwired: 11 in]
          n286 = call "BRig_dataMTrig_Laser_T_l1.vi"() -> ("output_Laser_T_l1"=w714:i32)  [unwired: 11 in]
          n287 = Index Array(array=w731, index #1=w713, index #2=w712, index #3=w715, index #4=w714) -> (element #1=w735:u16, element #2=w734:u16, element #3=w718:u16, element #4=w717:u16)
          n288 = Add(x=w716, y=w735) -> (x+y=w737:u16)
          n289 = Add(x=w716, y=w718) -> (x+y=w725:u16)
          n290 = Less?(x=w737, y=w734) -> (x < y?=w729:bool)
          n291 = Less?(x=w725, y=w717) -> (x < y?=w722:bool)
          n292 = Decrement(x=w727) -> (x-1=w738:u16)
          n293 = Decrement(x=w723) -> (x-1=w726:u16)
          n294 = Select(t=w737, s=w729, f=u16 0) -> (s? t:f=w733:u16)
          n295 = Select(t=w727, s=w729, f=w738) -> (s? t:f=w732:u16)
          n296 = Select(t=w725, s=w722, f=u16 0) -> (s? t:f=w720:u16)
          n297 = Select(t=w723, s=w722, f=w726) -> (s? t:f=w719:u16)
          n298 = Replace Array Subset(array=w731, new element #1=w733, index #1=w713, new element #2=w732, index #2=w728, new element #3=w720, index #3=w715, new element #4=w719, index #4=w721) -> (w730:u16[])
        }
        frame 13 {
          # "Audio_L"
          # "Tcycle"
          # "count"
          n299 = call "BRig_dataMTrig_CueLed_c.vi"() -> ("output_CueLed_c"=w742:i32)  [unwired: 11 in]
          n300 = call "BRig_dataMTrig_CueLed_T.vi"() -> ("output_CueLed_T"=w741:i32)  [unwired: 11 in]
          n301 = call "BRig_dataMTrig_Audio_c_L.vi"() -> ("output_Audio_c_L"=w746:i32)  [unwired: 11 in]
          n302 = call "BRig_dataMTrig_Audio_T_L.vi"() -> ("output_Audio_T_L"=w749:i32)  [unwired: 11 in]
          n303 = call "BRig_dataMTrig_Laser_c_l1.vi"() -> ("output_Laser_c_l1"=w740:i32)  [unwired: 11 in]
          n304 = call "BRig_dataMTrig_Laser_T_l1.vi"() -> ("output_Laser_T_l1"=w739:i32)  [unwired: 11 in]
          n305 = Index Array(array=w767, index #1=w746, index #2=w749, index #3=w742, index #4=w741, index #5=w740, index #6=w739) -> (element #1=w748:u16, element #2=w747:u16, element #3=w771:u16, element #4=w770:u16, element #5=w752:u16, element #6=w751:u16)
          n306 = Add(x=w750, y=w748) -> (x+y=w776:u16)
          n307 = Add(x=w750, y=w771) -> (x+y=w773:u16)
          n308 = Add(x=w750, y=w752) -> (x+y=w759:u16)
          n309 = Less?(x=w776, y=w747) -> (x < y?=w765:bool)
          n310 = Less?(x=w773, y=w770) -> (x < y?=w764:bool)
          n311 = Less?(x=w759, y=w751) -> (x < y?=w756:bool)
          n312 = Decrement(x=w763) -> (x-1=w777:u16)
          n313 = Decrement(x=w761) -> (x-1=w774:u16)
          n314 = Decrement(x=w757) -> (x-1=w760:u16)
          n315 = Select(t=w776, s=w765, f=u16 0) -> (s? t:f=w745:u16)
          n316 = Select(t=w763, s=w765, f=w777) -> (s? t:f=w743:u16)
          n317 = Select(t=w773, s=w764, f=u16 0) -> (s? t:f=w769:u16)
          n318 = Select(t=w761, s=w764, f=w774) -> (s? t:f=w768:u16)
          n319 = Select(t=w759, s=w756, f=u16 0) -> (s? t:f=w754:u16)
          n320 = Select(t=w757, s=w756, f=w760) -> (s? t:f=w753:u16)
          n321 = Replace Array Subset(array=w767, new element #1=w745, index #1=w746, new element #2=w743, index #2=w744, new element #3=w769, index #3=w742, new element #4=w768, index #4=w762, new element #5=w754, index #5=w740, new element #6=w753, index #6=w755) -> (w766:u16[])
        }
        frame 14 {
          # "Audio_R"
          # "Tcycle"
          # "count"
          n322 = call "BRig_dataMTrig_CueLed_c.vi"() -> ("output_CueLed_c"=w781:i32)  [unwired: 11 in]
          n323 = call "BRig_dataMTrig_CueLed_T.vi"() -> ("output_CueLed_T"=w780:i32)  [unwired: 11 in]
          n324 = call "BRig_dataMTrig_Laser_c_l1.vi"() -> ("output_Laser_c_l1"=w779:i32)  [unwired: 11 in]
          n325 = call "BRig_dataMTrig_Laser_T_l1.vi"() -> ("output_Laser_T_l1"=w778:i32)  [unwired: 11 in]
          n326 = call "BRig_dataMTrig_Audio_c_R.vi"() -> ("output_Audio_c_R"=w810:i32)  [unwired: 11 in]
          n327 = call "BRig_dataMTrig_Audio_T_R.vi"() -> ("output_Audio_T_R"=w811:i32)  [unwired: 11 in]
          n328 = Index Array(array=w800, index #1=w810, index #2=w811, index #3=w781, index #4=w780, index #5=w779, index #6=w778) -> (element #1=w813:u16, element #2=w812:u16, element #3=w804:u16, element #4=w803:u16, element #5=w784:u16, element #6=w783:u16)
          n329 = Add(x=w782, y=w813) -> (x+y=w815:u16)
          n330 = Add(x=w782, y=w804) -> (x+y=w806:u16)
          n331 = Add(x=w782, y=w784) -> (x+y=w791:u16)
          n332 = Less?(x=w815, y=w812) -> (x < y?=w798:bool)
          n333 = Less?(x=w806, y=w803) -> (x < y?=w797:bool)
          n334 = Less?(x=w791, y=w783) -> (x < y?=w788:bool)
          n335 = Decrement(x=w795) -> (x-1=w816:u16)
          n336 = Decrement(x=w793) -> (x-1=w807:u16)
          n337 = Decrement(x=w789) -> (x-1=w792:u16)
          n338 = Select(t=w815, s=w798, f=u16 0) -> (s? t:f=w809:u16)
          n339 = Select(t=w795, s=w798, f=w816) -> (s? t:f=w808:u16)
          n340 = Select(t=w806, s=w797, f=u16 0) -> (s? t:f=w802:u16)
          n341 = Select(t=w793, s=w797, f=w807) -> (s? t:f=w801:u16)
          n342 = Select(t=w791, s=w788, f=u16 0) -> (s? t:f=w786:u16)
          n343 = Select(t=w789, s=w788, f=w792) -> (s? t:f=w785:u16)
          n344 = Replace Array Subset(array=w800, new element #1=w809, index #1=w810, new element #2=w808, index #2=w796, new element #3=w802, index #3=w781, new element #4=w801, index #4=w794, new element #5=w786, index #5=w779, new element #6=w785, index #6=w787) -> (w799:u16[])
        }
        frame 15 {
          # "Audio_R"
          # "Tcycle"
          # "count"
          # "Audio_L"
          # "Tcycle"
          # "count"
          n345 = call "BRig_dataMTrig_Audio_c_L.vi"() -> ("output_Audio_c_L"=w859:i32)  [unwired: 11 in]
          n346 = call "BRig_dataMTrig_Audio_T_L.vi"() -> ("output_Audio_T_L"=w864:i32)  [unwired: 11 in]
          n347 = call "BRig_dataMTrig_Audio_c_R.vi"() -> ("output_Audio_c_R"=w852:i32)  [unwired: 11 in]
          n348 = call "BRig_dataMTrig_Audio_T_R.vi"() -> ("output_Audio_T_R"=w853:i32)  [unwired: 11 in]
          n349 = call "BRig_dataMTrig_CueLed_c.vi"() -> ("output_CueLed_c"=w820:i32)  [unwired: 11 in]
          n350 = call "BRig_dataMTrig_CueLed_T.vi"() -> ("output_CueLed_T"=w819:i32)  [unwired: 11 in]
          n351 = call "BRig_dataMTrig_Laser_c_l1.vi"() -> ("output_Laser_c_l1"=w818:i32)  [unwired: 11 in]
          n352 = call "BRig_dataMTrig_Laser_T_l1.vi"() -> ("output_Laser_T_l1"=w817:i32)  [unwired: 11 in]
          n353 = Index Array(array=w842, index #1=w859, index #2=w864, index #3=w852, index #4=w853, index #5=w820, index #6=w819, index #7=w818, index #8=w817) -> (element #1=w863:u16, element #2=w862:u16, element #3=w855:u16, element #4=w854:u16, element #5=w846:u16, element #6=w845:u16, element #7=w823:u16, element #8=w822:u16)
          n354 = Add(x=w821, y=w863) -> (x+y=w866:u16)
          n355 = Add(x=w821, y=w855) -> (x+y=w857:u16)
          n356 = Add(x=w821, y=w846) -> (x+y=w848:u16)
          n357 = Add(x=w821, y=w823) -> (x+y=w830:u16)
          n358 = Less?(x=w866, y=w862) -> (x < y?=w840:bool)
          n359 = Less?(x=w857, y=w854) -> (x < y?=w839:bool)
          n360 = Less?(x=w848, y=w845) -> (x < y?=w838:bool)
          n361 = Less?(x=w830, y=w822) -> (x < y?=w827:bool)
          n362 = Decrement(x=w836) -> (x-1=w867:u16)
          n363 = Decrement(x=w834) -> (x-1=w858:u16)
          n364 = Decrement(x=w832) -> (x-1=w849:u16)
          n365 = Decrement(x=w828) -> (x-1=w831:u16)
          n366 = Select(t=w866, s=w840, f=u16 0) -> (s? t:f=w861:u16)
          n367 = Select(t=w836, s=w840, f=w867) -> (s? t:f=w860:u16)
          n368 = Select(t=w857, s=w839, f=u16 0) -> (s? t:f=w851:u16)
          n369 = Select(t=w834, s=w839, f=w858) -> (s? t:f=w850:u16)
          n370 = Select(t=w848, s=w838, f=u16 0) -> (s? t:f=w844:u16)
          n371 = Select(t=w832, s=w838, f=w849) -> (s? t:f=w843:u16)
          n372 = Select(t=w830, s=w827, f=u16 0) -> (s? t:f=w825:u16)
          n373 = Select(t=w828, s=w827, f=w831) -> (s? t:f=w824:u16)
          n374 = Replace Array Subset(array=w842, new element #1=w861, index #1=w859, new element #2=w860, index #2=w837, new element #3=w851, index #3=w852, new element #4=w850, index #4=w835, new element #5=w844, index #5=w820, new element #6=w843, index #6=w833, new element #7=w825, index #7=w818, new element #8=w824, index #8=w826) -> (w841:u16[])
        }
        frame 16 {
          n375 = call "BRig_dataMTrig_Laser_c_l2.vi"() -> ("output_Laser_c_l2"=w869:i32)  [unwired: 11 in]
          n376 = call "BRig_dataMTrig_Laser_T_l2.vi"() -> ("output_Laser_T_l2"=w868:i32)  [unwired: 11 in]
          n377 = Index Array(array=w882, index #1=w869, index #2=w868) -> (element #1=w876:u16, element #2=w875:u16)
          n378 = Add(x=w874, y=w876) -> (x+y=w879:u16)
          n379 = Less?(x=w879, y=w875) -> (x < y?=w870:bool)
          n380 = Decrement(x=w877) -> (x-1=w880:u16)
          n381 = Select(t=w879, s=w870, f=u16 0) -> (s? t:f=w873:u16)
          n382 = Select(t=w877, s=w870, f=w880) -> (s? t:f=w871:u16)
          n383 = Replace Array Subset(array=w882, new element #1=w873, index #1=w869, new element #2=w871, index #2=w872) -> (w881:u16[])
        }
        frame 17 {
          # "Audio_L"
          # "Tcycle"
          # "count"
          n384 = call "BRig_dataMTrig_Audio_c_L.vi"() -> ("output_Audio_c_L"=w901:i32)  [unwired: 11 in]
          n385 = call "BRig_dataMTrig_Audio_T_L.vi"() -> ("output_Audio_T_L"=w906:i32)  [unwired: 11 in]
          n386 = call "BRig_dataMTrig_Laser_c_l2.vi"() -> ("output_Laser_c_l2"=w884:i32)  [unwired: 11 in]
          n387 = call "BRig_dataMTrig_Laser_T_l2.vi"() -> ("output_Laser_T_l2"=w883:i32)  [unwired: 11 in]
          n388 = Index Array(array=w900, index #1=w901, index #2=w906, index #3=w884, index #4=w883) -> (element #1=w905:u16, element #2=w904:u16, element #3=w886:u16, element #4=w885:u16)
          n389 = Add(x=w891, y=w905) -> (x+y=w908:u16)
          n390 = Add(x=w891, y=w886) -> (x+y=w894:u16)
          n391 = Less?(x=w908, y=w904) -> (x < y?=w898:bool)
          n392 = Less?(x=w894, y=w885) -> (x < y?=w890:bool)
          n393 = Decrement(x=w896) -> (x-1=w909:u16)
          n394 = Decrement(x=w892) -> (x-1=w895:u16)
          n395 = Select(t=w908, s=w898, f=u16 0) -> (s? t:f=w903:u16)
          n396 = Select(t=w896, s=w898, f=w909) -> (s? t:f=w902:u16)
          n397 = Select(t=w894, s=w890, f=u16 0) -> (s? t:f=w889:u16)
          n398 = Select(t=w892, s=w890, f=w895) -> (s? t:f=w887:u16)
          n399 = Replace Array Subset(array=w900, new element #1=w903, index #1=w901, new element #2=w902, index #2=w897, new element #3=w889, index #3=w884, new element #4=w887, index #4=w888) -> (w899:u16[])
        }
        frame 18 {
          # "Audio_R"
          # "Tcycle"
          # "count"
          n400 = call "BRig_dataMTrig_Laser_c_l2.vi"() -> ("output_Laser_c_l2"=w911:i32)  [unwired: 11 in]
          n401 = call "BRig_dataMTrig_Laser_T_l2.vi"() -> ("output_Laser_T_l2"=w910:i32)  [unwired: 11 in]
          n402 = call "BRig_dataMTrig_Audio_c_R.vi"() -> ("output_Audio_c_R"=w930:i32)  [unwired: 11 in]
          n403 = call "BRig_dataMTrig_Audio_T_R.vi"() -> ("output_Audio_T_R"=w931:i32)  [unwired: 11 in]
          n404 = Index Array(array=w927, index #1=w930, index #2=w931, index #3=w911, index #4=w910) -> (element #1=w933:u16, element #2=w932:u16, element #3=w913:u16, element #4=w912:u16)
          n405 = Add(x=w918, y=w933) -> (x+y=w935:u16)
          n406 = Add(x=w918, y=w913) -> (x+y=w921:u16)
          n407 = Less?(x=w935, y=w932) -> (x < y?=w925:bool)
          n408 = Less?(x=w921, y=w912) -> (x < y?=w917:bool)
          n409 = Decrement(x=w923) -> (x-1=w936:u16)
          n410 = Decrement(x=w919) -> (x-1=w922:u16)
          n411 = Select(t=w935, s=w925, f=u16 0) -> (s? t:f=w929:u16)
          n412 = Select(t=w923, s=w925, f=w936) -> (s? t:f=w928:u16)
          n413 = Select(t=w921, s=w917, f=u16 0) -> (s? t:f=w916:u16)
          n414 = Select(t=w919, s=w917, f=w922) -> (s? t:f=w914:u16)
          n415 = Replace Array Subset(array=w927, new element #1=w929, index #1=w930, new element #2=w928, index #2=w924, new element #3=w916, index #3=w911, new element #4=w914, index #4=w915) -> (w926:u16[])
        }
        frame 19 {
          # "Audio_R"
          # "Tcycle"
          # "count"
          # "Audio_L"
          # "Tcycle"
          # "count"
          n416 = call "BRig_dataMTrig_Audio_c_L.vi"() -> ("output_Audio_c_L"=w967:i32)  [unwired: 11 in]
          n417 = call "BRig_dataMTrig_Audio_T_L.vi"() -> ("output_Audio_T_L"=w972:i32)  [unwired: 11 in]
          n418 = call "BRig_dataMTrig_Laser_c_l2.vi"() -> ("output_Laser_c_l2"=w938:i32)  [unwired: 11 in]
          n419 = call "BRig_dataMTrig_Laser_T_l2.vi"() -> ("output_Laser_T_l2"=w937:i32)  [unwired: 11 in]
          n420 = call "BRig_dataMTrig_Audio_c_R.vi"() -> ("output_Audio_c_R"=w960:i32)  [unwired: 11 in]
          n421 = call "BRig_dataMTrig_Audio_T_R.vi"() -> ("output_Audio_T_R"=w961:i32)  [unwired: 11 in]
          n422 = Index Array(array=w957, index #1=w967, index #2=w972, index #3=w960, index #4=w961, index #5=w938, index #6=w937) -> (element #1=w971:u16, element #2=w970:u16, element #3=w963:u16, element #4=w962:u16, element #5=w943:u16, element #6=w942:u16)
          n423 = Add(x=w945, y=w971) -> (x+y=w974:u16)
          n424 = Add(x=w945, y=w963) -> (x+y=w965:u16)
          n425 = Add(x=w945, y=w943) -> (x+y=w948:u16)
          n426 = Less?(x=w974, y=w970) -> (x < y?=w955:bool)
          n427 = Less?(x=w965, y=w962) -> (x < y?=w954:bool)
          n428 = Less?(x=w948, y=w942) -> (x < y?=w944:bool)
          n429 = Decrement(x=w952) -> (x-1=w975:u16)
          n430 = Decrement(x=w950) -> (x-1=w966:u16)
          n431 = Decrement(x=w946) -> (x-1=w949:u16)
          n432 = Select(t=w974, s=w955, f=u16 0) -> (s? t:f=w969:u16)
          n433 = Select(t=w952, s=w955, f=w975) -> (s? t:f=w968:u16)
          n434 = Select(t=w965, s=w954, f=u16 0) -> (s? t:f=w959:u16)
          n435 = Select(t=w950, s=w954, f=w966) -> (s? t:f=w958:u16)
          n436 = Select(t=w948, s=w944, f=u16 0) -> (s? t:f=w941:u16)
          n437 = Select(t=w946, s=w944, f=w949) -> (s? t:f=w939:u16)
          n438 = Replace Array Subset(array=w957, new element #1=w969, index #1=w967, new element #2=w968, index #2=w953, new element #3=w959, index #3=w960, new element #4=w958, index #4=w951, new element #5=w941, index #5=w938, new element #6=w939, index #6=w940) -> (w956:u16[])
        }
        frame 20 {
          n439 = call "BRig_dataMTrig_CueLed_c.vi"() -> ("output_CueLed_c"=w990:i32)  [unwired: 11 in]
          n440 = call "BRig_dataMTrig_CueLed_T.vi"() -> ("output_CueLed_T"=w989:i32)  [unwired: 11 in]
          n441 = call "BRig_dataMTrig_Laser_c_l2.vi"() -> ("output_Laser_c_l2"=w977:i32)  [unwired: 11 in]
          n442 = call "BRig_dataMTrig_Laser_T_l2.vi"() -> ("output_Laser_T_l2"=w976:i32)  [unwired: 11 in]
          n443 = Index Array(array=w995, index #1=w990, index #2=w989, index #3=w977, index #4=w976) -> (element #1=w999:u16, element #2=w998:u16, element #3=w982:u16, element #4=w981:u16)
          n444 = Add(x=w984, y=w999) -> (x+y=w1001:u16)
          n445 = Add(x=w984, y=w982) -> (x+y=w987:u16)
          n446 = Less?(x=w1001, y=w998) -> (x < y?=w993:bool)
          n447 = Less?(x=w987, y=w981) -> (x < y?=w983:bool)
          n448 = Decrement(x=w991) -> (x-1=w1002:u16)
          n449 = Decrement(x=w985) -> (x-1=w988:u16)
          n450 = Select(t=w1001, s=w993, f=u16 0) -> (s? t:f=w997:u16)
          n451 = Select(t=w991, s=w993, f=w1002) -> (s? t:f=w996:u16)
          n452 = Select(t=w987, s=w983, f=u16 0) -> (s? t:f=w980:u16)
          n453 = Select(t=w985, s=w983, f=w988) -> (s? t:f=w978:u16)
          n454 = Replace Array Subset(array=w995, new element #1=w997, index #1=w990, new element #2=w996, index #2=w992, new element #3=w980, index #3=w977, new element #4=w978, index #4=w979) -> (w994:u16[])
        }
        frame 21 {
          # "Audio_L"
          # "Tcycle"
          # "count"
          n455 = call "BRig_dataMTrig_Audio_c_L.vi"() -> ("output_Audio_c_L"=w1033:i32)  [unwired: 11 in]
          n456 = call "BRig_dataMTrig_Audio_T_L.vi"() -> ("output_Audio_T_L"=w1038:i32)  [unwired: 11 in]
          n457 = call "BRig_dataMTrig_CueLed_c.vi"() -> ("output_CueLed_c"=w1010:i32)  [unwired: 11 in]
          n458 = call "BRig_dataMTrig_CueLed_T.vi"() -> ("output_CueLed_T"=w1009:i32)  [unwired: 11 in]
          n459 = call "BRig_dataMTrig_Laser_c_l2.vi"() -> ("output_Laser_c_l2"=w1004:i32)  [unwired: 11 in]
          n460 = call "BRig_dataMTrig_Laser_T_l2.vi"() -> ("output_Laser_T_l2"=w1003:i32)  [unwired: 11 in]
          n461 = Index Array(array=w1029, index #1=w1033, index #2=w1038, index #3=w1010, index #4=w1009, index #5=w1004, index #6=w1003) -> (element #1=w1037:u16, element #2=w1036:u16, element #3=w1008:u16, element #4=w1007:u16, element #5=w1006:u16, element #6=w1005:u16)
          n462 = Add(x=w1018, y=w1037) -> (x+y=w1040:u16)
          n463 = Add(x=w1018, y=w1008) -> (x+y=w1031:u16)
          n464 = Add(x=w1018, y=w1006) -> (x+y=w1021:u16)
          n465 = Less?(x=w1040, y=w1036) -> (x < y?=w1027:bool)
          n466 = Less?(x=w1031, y=w1007) -> (x < y?=w1026:bool)
          n467 = Less?(x=w1021, y=w1005) -> (x < y?=w1017:bool)
          n468 = Decrement(x=w1024) -> (x-1=w1041:u16)
          n469 = Decrement(x=w1023) -> (x-1=w1032:u16)
          n470 = Decrement(x=w1019) -> (x-1=w1022:u16)
          n471 = Select(t=w1040, s=w1027, f=u16 0) -> (s? t:f=w1035:u16)
          n472 = Select(t=w1024, s=w1027, f=w1041) -> (s? t:f=w1034:u16)
          n473 = Select(t=w1031, s=w1026, f=u16 0) -> (s? t:f=w1016:u16)
          n474 = Select(t=w1023, s=w1026, f=w1032) -> (s? t:f=w1014:u16)
          n475 = Select(t=w1021, s=w1017, f=u16 0) -> (s? t:f=w1013:u16)
          n476 = Select(t=w1019, s=w1017, f=w1022) -> (s? t:f=w1011:u16)
          n477 = Replace Array Subset(array=w1029, new element #1=w1035, index #1=w1033, new element #2=w1034, index #2=w1025, new element #3=w1016, index #3=w1010, new element #4=w1014, index #4=w1015, new element #5=w1013, index #5=w1004, new element #6=w1011, index #6=w1012) -> (w1028:u16[])
        }
        frame 22 {
          # "Audio_R"
          # "Tcycle"
          # "count"
          n478 = call "BRig_dataMTrig_Audio_c_R.vi"() -> ("output_Audio_c_R"=w1074:i32)  [unwired: 11 in]
          n479 = call "BRig_dataMTrig_Audio_T_R.vi"() -> ("output_Audio_T_R"=w1075:i32)  [unwired: 11 in]
          n480 = call "BRig_dataMTrig_CueLed_c.vi"() -> ("output_CueLed_c"=w1056:i32)  [unwired: 11 in]
          n481 = call "BRig_dataMTrig_CueLed_T.vi"() -> ("output_CueLed_T"=w1055:i32)  [unwired: 11 in]
          n482 = call "BRig_dataMTrig_Laser_c_l2.vi"() -> ("output_Laser_c_l2"=w1043:i32)  [unwired: 11 in]
          n483 = call "BRig_dataMTrig_Laser_T_l2.vi"() -> ("output_Laser_T_l2"=w1042:i32)  [unwired: 11 in]
          n484 = Index Array(array=w1064, index #1=w1074, index #2=w1075, index #3=w1056, index #4=w1055, index #5=w1043, index #6=w1042) -> (element #1=w1077:u16, element #2=w1076:u16, element #3=w1068:u16, element #4=w1067:u16, element #5=w1045:u16, element #6=w1044:u16)
          n485 = Add(x=w1050, y=w1077) -> (x+y=w1079:u16)
          n486 = Add(x=w1050, y=w1068) -> (x+y=w1070:u16)
          n487 = Add(x=w1050, y=w1045) -> (x+y=w1053:u16)
          n488 = Less?(x=w1079, y=w1076) -> (x < y?=w1062:bool)
          n489 = Less?(x=w1070, y=w1067) -> (x < y?=w1061:bool)
          n490 = Less?(x=w1053, y=w1044) -> (x < y?=w1049:bool)
          n491 = Decrement(x=w1059) -> (x-1=w1080:u16)
          n492 = Decrement(x=w1057) -> (x-1=w1071:u16)
          n493 = Decrement(x=w1051) -> (x-1=w1054:u16)
          n494 = Select(t=w1079, s=w1062, f=u16 0) -> (s? t:f=w1073:u16)
          n495 = Select(t=w1059, s=w1062, f=w1080) -> (s? t:f=w1072:u16)
          n496 = Select(t=w1070, s=w1061, f=u16 0) -> (s? t:f=w1066:u16)
          n497 = Select(t=w1057, s=w1061, f=w1071) -> (s? t:f=w1065:u16)
          n498 = Select(t=w1053, s=w1049, f=u16 0) -> (s? t:f=w1048:u16)
          n499 = Select(t=w1051, s=w1049, f=w1054) -> (s? t:f=w1046:u16)
          n500 = Replace Array Subset(array=w1064, new element #1=w1073, index #1=w1074, new element #2=w1072, index #2=w1060, new element #3=w1066, index #3=w1056, new element #4=w1065, index #4=w1058, new element #5=w1048, index #5=w1043, new element #6=w1046, index #6=w1047) -> (w1063:u16[])
        }
        frame 23 {
          # "Audio_R"
          # "Tcycle"
          # "count"
          # "Audio_L"
          # "Tcycle"
          # "count"
          n501 = call "BRig_dataMTrig_Audio_c_L.vi"() -> ("output_Audio_c_L"=w1123:i32)  [unwired: 11 in]
          n502 = call "BRig_dataMTrig_Audio_T_L.vi"() -> ("output_Audio_T_L"=w1128:i32)  [unwired: 11 in]
          n503 = call "BRig_dataMTrig_Audio_c_R.vi"() -> ("output_Audio_c_R"=w1116:i32)  [unwired: 11 in]
          n504 = call "BRig_dataMTrig_Audio_T_R.vi"() -> ("output_Audio_T_R"=w1117:i32)  [unwired: 11 in]
          n505 = call "BRig_dataMTrig_CueLed_c.vi"() -> ("output_CueLed_c"=w1095:i32)  [unwired: 11 in]
          n506 = call "BRig_dataMTrig_CueLed_T.vi"() -> ("output_CueLed_T"=w1094:i32)  [unwired: 11 in]
          n507 = call "BRig_dataMTrig_Laser_c_l2.vi"() -> ("output_Laser_c_l2"=w1082:i32)  [unwired: 11 in]
          n508 = call "BRig_dataMTrig_Laser_T_l2.vi"() -> ("output_Laser_T_l2"=w1081:i32)  [unwired: 11 in]
          n509 = Index Array(array=w1106, index #1=w1123, index #2=w1128, index #3=w1116, index #4=w1117, index #5=w1095, index #6=w1094, index #7=w1082, index #8=w1081) -> (element #1=w1127:u16, element #2=w1126:u16, element #3=w1119:u16, element #4=w1118:u16, element #5=w1110:u16, element #6=w1109:u16, element #7=w1084:u16, element #8=w1083:u16)
          n510 = Add(x=w1089, y=w1127) -> (x+y=w1130:u16)
          n511 = Add(x=w1089, y=w1119) -> (x+y=w1121:u16)
          n512 = Add(x=w1089, y=w1110) -> (x+y=w1112:u16)
          n513 = Add(x=w1089, y=w1084) -> (x+y=w1092:u16)
          n514 = Less?(x=w1130, y=w1126) -> (x < y?=w1104:bool)
          n515 = Less?(x=w1121, y=w1118) -> (x < y?=w1103:bool)
          n516 = Less?(x=w1112, y=w1109) -> (x < y?=w1102:bool)
          n517 = Less?(x=w1092, y=w1083) -> (x < y?=w1088:bool)
          n518 = Decrement(x=w1100) -> (x-1=w1131:u16)
          n519 = Decrement(x=w1098) -> (x-1=w1122:u16)
          n520 = Decrement(x=w1096) -> (x-1=w1113:u16)
          n521 = Decrement(x=w1090) -> (x-1=w1093:u16)
          n522 = Select(t=w1130, s=w1104, f=u16 0) -> (s? t:f=w1125:u16)
          n523 = Select(t=w1100, s=w1104, f=w1131) -> (s? t:f=w1124:u16)
          n524 = Select(t=w1121, s=w1103, f=u16 0) -> (s? t:f=w1115:u16)
          n525 = Select(t=w1098, s=w1103, f=w1122) -> (s? t:f=w1114:u16)
          n526 = Select(t=w1112, s=w1102, f=u16 0) -> (s? t:f=w1108:u16)
          n527 = Select(t=w1096, s=w1102, f=w1113) -> (s? t:f=w1107:u16)
          n528 = Select(t=w1092, s=w1088, f=u16 0) -> (s? t:f=w1087:u16)
          n529 = Select(t=w1090, s=w1088, f=w1093) -> (s? t:f=w1085:u16)
          n530 = Replace Array Subset(array=w1106, new element #1=w1125, index #1=w1123, new element #2=w1124, index #2=w1101, new element #3=w1115, index #3=w1116, new element #4=w1114, index #4=w1099, new element #5=w1108, index #5=w1095, new element #6=w1107, index #6=w1097, new element #7=w1087, index #7=w1082, new element #8=w1085, index #8=w1086) -> (w1105:u16[])
        }
        frame 24 {
          n531 = call "BRig_dataMTrig_Laser_c_l2.vi"() -> ("output_Laser_c_l2"=w1133:i32)  [unwired: 11 in]
          n532 = call "BRig_dataMTrig_Laser_T_l2.vi"() -> ("output_Laser_T_l2"=w1132:i32)  [unwired: 11 in]
          n533 = call "BRig_dataMTrig_Laser_c_l1.vi"() -> ("output_Laser_c_l1"=w1146:i32)  [unwired: 11 in]
          n534 = call "BRig_dataMTrig_Laser_T_l1.vi"() -> ("output_Laser_T_l1"=w1145:i32)  [unwired: 11 in]
          n535 = Index Array(array=w1158, index #1=w1146, index #2=w1145, index #3=w1133, index #4=w1132) -> (element #1=w1148:u16, element #2=w1147:u16, element #3=w1140:u16, element #4=w1139:u16)
          n536 = Add(x=w1138, y=w1148) -> (x+y=w1155:u16)
          n537 = Add(x=w1138, y=w1140) -> (x+y=w1143:u16)
          n538 = Less?(x=w1155, y=w1147) -> (x < y?=w1152:bool)
          n539 = Less?(x=w1143, y=w1139) -> (x < y?=w1134:bool)
          n540 = Decrement(x=w1153) -> (x-1=w1156:u16)
          n541 = Decrement(x=w1141) -> (x-1=w1144:u16)
          n542 = Select(t=w1155, s=w1152, f=u16 0) -> (s? t:f=w1150:u16)
          n543 = Select(t=w1153, s=w1152, f=w1156) -> (s? t:f=w1149:u16)
          n544 = Select(t=w1143, s=w1134, f=u16 0) -> (s? t:f=w1137:u16)
          n545 = Select(t=w1141, s=w1134, f=w1144) -> (s? t:f=w1135:u16)
          n546 = Replace Array Subset(array=w1158, new element #1=w1150, index #1=w1146, new element #2=w1149, index #2=w1151, new element #3=w1137, index #3=w1133, new element #4=w1135, index #4=w1136) -> (w1157:u16[])
        }
        frame 25 {
          # "Audio_L"
          # "Tcycle"
          # "count"
          n547 = call "BRig_dataMTrig_Audio_c_L.vi"() -> ("output_Audio_c_L"=w1164:i32)  [unwired: 11 in]
          n548 = call "BRig_dataMTrig_Audio_T_L.vi"() -> ("output_Audio_T_L"=w1167:i32)  [unwired: 11 in]
          n549 = call "BRig_dataMTrig_Laser_c_l2.vi"() -> ("output_Laser_c_l2"=w1160:i32)  [unwired: 11 in]
          n550 = call "BRig_dataMTrig_Laser_T_l2.vi"() -> ("output_Laser_T_l2"=w1159:i32)  [unwired: 11 in]
          n551 = call "BRig_dataMTrig_Laser_c_l1.vi"() -> ("output_Laser_c_l1"=w1180:i32)  [unwired: 11 in]
          n552 = call "BRig_dataMTrig_Laser_T_l1.vi"() -> ("output_Laser_T_l1"=w1179:i32)  [unwired: 11 in]
          n553 = Index Array(array=w1194, index #1=w1164, index #2=w1167, index #3=w1180, index #4=w1179, index #5=w1160, index #6=w1159) -> (element #1=w1166:u16, element #2=w1165:u16, element #3=w1182:u16, element #4=w1181:u16, element #5=w1174:u16, element #6=w1173:u16)
          n554 = Add(x=w1172, y=w1166) -> (x+y=w1196:u16)
          n555 = Add(x=w1172, y=w1182) -> (x+y=w1189:u16)
          n556 = Add(x=w1172, y=w1174) -> (x+y=w1177:u16)
          n557 = Less?(x=w1196, y=w1165) -> (x < y?=w1192:bool)
          n558 = Less?(x=w1189, y=w1181) -> (x < y?=w1186:bool)
          n559 = Less?(x=w1177, y=w1173) -> (x < y?=w1168:bool)
          n560 = Decrement(x=w1191) -> (x-1=w1197:u16)
          n561 = Decrement(x=w1187) -> (x-1=w1190:u16)
          n562 = Decrement(x=w1175) -> (x-1=w1178:u16)
          n563 = Select(t=w1196, s=w1192, f=u16 0) -> (s? t:f=w1163:u16)
          n564 = Select(t=w1191, s=w1192, f=w1197) -> (s? t:f=w1161:u16)
          n565 = Select(t=w1189, s=w1186, f=u16 0) -> (s? t:f=w1184:u16)
          n566 = Select(t=w1187, s=w1186, f=w1190) -> (s? t:f=w1183:u16)
          n567 = Select(t=w1177, s=w1168, f=u16 0) -> (s? t:f=w1171:u16)
          n568 = Select(t=w1175, s=w1168, f=w1178) -> (s? t:f=w1169:u16)
          n569 = Replace Array Subset(array=w1194, new element #1=w1163, index #1=w1164, new element #2=w1161, index #2=w1162, new element #3=w1184, index #3=w1180, new element #4=w1183, index #4=w1185, new element #5=w1171, index #5=w1160, new element #6=w1169, index #6=w1170) -> (w1193:u16[])
        }
        frame 26 {
          # "Audio_R"
          # "Tcycle"
          # "count"
          n570 = call "BRig_dataMTrig_Audio_c_R.vi"() -> ("output_Audio_c_R"=w1200:i32)  [unwired: 11 in]
          n571 = call "BRig_dataMTrig_Audio_T_R.vi"() -> ("output_Audio_T_R"=w1206:i32)  [unwired: 11 in]
          n572 = call "BRig_dataMTrig_Laser_c_l1.vi"() -> ("output_Laser_c_l1"=w1219:i32)  [unwired: 11 in]
          n573 = call "BRig_dataMTrig_Laser_T_l1.vi"() -> ("output_Laser_T_l1"=w1218:i32)  [unwired: 11 in]
          n574 = call "BRig_dataMTrig_Laser_c_l2.vi"() -> ("output_Laser_c_l2"=w1199:i32)  [unwired: 11 in]
          n575 = call "BRig_dataMTrig_Laser_T_l2.vi"() -> ("output_Laser_T_l2"=w1198:i32)  [unwired: 11 in]
          n576 = Index Array(array=w1233, index #1=w1200, index #2=w1206, index #3=w1219, index #4=w1218, index #5=w1199, index #6=w1198) -> (element #1=w1204:u16, element #2=w1205:u16, element #3=w1221:u16, element #4=w1220:u16, element #5=w1213:u16, element #6=w1212:u16)
          n577 = Add(x=w1211, y=w1204) -> (x+y=w1235:u16)
          n578 = Add(x=w1211, y=w1221) -> (x+y=w1228:u16)
          n579 = Add(x=w1211, y=w1213) -> (x+y=w1216:u16)
          n580 = Less?(x=w1235, y=w1205) -> (x < y?=w1231:bool)
          n581 = Less?(x=w1228, y=w1220) -> (x < y?=w1225:bool)
          n582 = Less?(x=w1216, y=w1212) -> (x < y?=w1207:bool)
          n583 = Decrement(x=w1230) -> (x-1=w1236:u16)
          n584 = Decrement(x=w1226) -> (x-1=w1229:u16)
          n585 = Decrement(x=w1214) -> (x-1=w1217:u16)
          n586 = Select(t=w1235, s=w1231, f=u16 0) -> (s? t:f=w1201:u16)
          n587 = Select(t=w1230, s=w1231, f=w1236) -> (s? t:f=w1203:u16)
          n588 = Select(t=w1228, s=w1225, f=u16 0) -> (s? t:f=w1223:u16)
          n589 = Select(t=w1226, s=w1225, f=w1229) -> (s? t:f=w1222:u16)
          n590 = Select(t=w1216, s=w1207, f=u16 0) -> (s? t:f=w1210:u16)
          n591 = Select(t=w1214, s=w1207, f=w1217) -> (s? t:f=w1208:u16)
          n592 = Replace Array Subset(array=w1233, new element #1=w1201, index #1=w1200, new element #2=w1203, index #2=w1202, new element #3=w1223, index #3=w1219, new element #4=w1222, index #4=w1224, new element #5=w1210, index #5=w1199, new element #6=w1208, index #6=w1209) -> (w1232:u16[])
        }
        frame 27 {
          # "Audio_R"
          # "Tcycle"
          # "count"
          # "Audio_L"
          # "Tcycle"
          # "count"
          n593 = call "BRig_dataMTrig_Audio_c_L.vi"() -> ("output_Audio_c_L"=w1239:i32)  [unwired: 11 in]
          n594 = call "BRig_dataMTrig_Audio_T_L.vi"() -> ("output_Audio_T_L"=w1251:i32)  [unwired: 11 in]
          n595 = call "BRig_dataMTrig_Audio_c_R.vi"() -> ("output_Audio_c_R"=w1243:i32)  [unwired: 11 in]
          n596 = call "BRig_dataMTrig_Audio_T_R.vi"() -> ("output_Audio_T_R"=w1252:i32)  [unwired: 11 in]
          n597 = call "BRig_dataMTrig_Laser_c_l1.vi"() -> ("output_Laser_c_l1"=w1265:i32)  [unwired: 11 in]
          n598 = call "BRig_dataMTrig_Laser_T_l1.vi"() -> ("output_Laser_T_l1"=w1264:i32)  [unwired: 11 in]
          n599 = call "BRig_dataMTrig_Laser_c_l2.vi"() -> ("output_Laser_c_l2"=w1238:i32)  [unwired: 11 in]
          n600 = call "BRig_dataMTrig_Laser_T_l2.vi"() -> ("output_Laser_T_l2"=w1237:i32)  [unwired: 11 in]
          n601 = Index Array(array=w1281, index #1=w1239, index #2=w1251, index #3=w1243, index #4=w1252, index #5=w1265, index #6=w1264, index #7=w1238, index #8=w1237) -> (element #1=w1247:u16, element #2=w1248:u16, element #3=w1249:u16, element #4=w1250:u16, element #5=w1267:u16, element #6=w1266:u16, element #7=w1259:u16, element #8=w1258:u16)
          n602 = Add(x=w1257, y=w1247) -> (x+y=w1286:u16)
          n603 = Add(x=w1257, y=w1249) -> (x+y=w1283:u16)
          n604 = Add(x=w1257, y=w1267) -> (x+y=w1274:u16)
          n605 = Add(x=w1257, y=w1259) -> (x+y=w1262:u16)
          n606 = Less?(x=w1286, y=w1248) -> (x < y?=w1279:bool)
          n607 = Less?(x=w1283, y=w1250) -> (x < y?=w1278:bool)
          n608 = Less?(x=w1274, y=w1266) -> (x < y?=w1271:bool)
          n609 = Less?(x=w1262, y=w1258) -> (x < y?=w1253:bool)
          n610 = Decrement(x=w1277) -> (x-1=w1287:u16)
          n611 = Decrement(x=w1276) -> (x-1=w1284:u16)
          n612 = Decrement(x=w1272) -> (x-1=w1275:u16)
          n613 = Decrement(x=w1260) -> (x-1=w1263:u16)
          n614 = Select(t=w1286, s=w1279, f=u16 0) -> (s? t:f=w1240:u16)
          n615 = Select(t=w1277, s=w1279, f=w1287) -> (s? t:f=w1242:u16)
          n616 = Select(t=w1283, s=w1278, f=u16 0) -> (s? t:f=w1244:u16)
          n617 = Select(t=w1276, s=w1278, f=w1284) -> (s? t:f=w1246:u16)
          n618 = Select(t=w1274, s=w1271, f=u16 0) -> (s? t:f=w1269:u16)
          n619 = Select(t=w1272, s=w1271, f=w1275) -> (s? t:f=w1268:u16)
          n620 = Select(t=w1262, s=w1253, f=u16 0) -> (s? t:f=w1256:u16)
          n621 = Select(t=w1260, s=w1253, f=w1263) -> (s? t:f=w1254:u16)
          n622 = Replace Array Subset(array=w1281, new element #1=w1240, index #1=w1239, new element #2=w1242, index #2=w1241, new element #3=w1244, index #3=w1243, new element #4=w1246, index #4=w1245, new element #5=w1269, index #5=w1265, new element #6=w1268, index #6=w1270, new element #7=w1256, index #7=w1238, new element #8=w1254, index #8=w1255) -> (w1280:u16[])
        }
        frame 28 {
          n623 = call "BRig_dataMTrig_CueLed_c.vi"() -> ("output_CueLed_c"=w1304:i32)  [unwired: 11 in]
          n624 = call "BRig_dataMTrig_CueLed_T.vi"() -> ("output_CueLed_T"=w1303:i32)  [unwired: 11 in]
          n625 = call "BRig_dataMTrig_Laser_c_l2.vi"() -> ("output_Laser_c_l2"=w1289:i32)  [unwired: 11 in]
          n626 = call "BRig_dataMTrig_Laser_T_l2.vi"() -> ("output_Laser_T_l2"=w1288:i32)  [unwired: 11 in]
          n627 = call "BRig_dataMTrig_Laser_c_l1.vi"() -> ("output_Laser_c_l1"=w1302:i32)  [unwired: 11 in]
          n628 = call "BRig_dataMTrig_Laser_T_l1.vi"() -> ("output_Laser_T_l1"=w1301:i32)  [unwired: 11 in]
          n629 = Index Array(array=w1319, index #1=w1304, index #2=w1303, index #3=w1302, index #4=w1301, index #5=w1289, index #6=w1288) -> (element #1=w1323:u16, element #2=w1322:u16, element #3=w1306:u16, element #4=w1305:u16, element #5=w1296:u16, element #6=w1295:u16)
          n630 = Add(x=w1294, y=w1323) -> (x+y=w1325:u16)
          n631 = Add(x=w1294, y=w1306) -> (x+y=w1313:u16)
          n632 = Add(x=w1294, y=w1296) -> (x+y=w1299:u16)
          n633 = Less?(x=w1325, y=w1322) -> (x < y?=w1317:bool)
          n634 = Less?(x=w1313, y=w1305) -> (x < y?=w1310:bool)
          n635 = Less?(x=w1299, y=w1295) -> (x < y?=w1290:bool)
          n636 = Decrement(x=w1315) -> (x-1=w1326:u16)
          n637 = Decrement(x=w1311) -> (x-1=w1314:u16)
          n638 = Decrement(x=w1297) -> (x-1=w1300:u16)
          n639 = Select(t=w1325, s=w1317, f=u16 0) -> (s? t:f=w1321:u16)
          n640 = Select(t=w1315, s=w1317, f=w1326) -> (s? t:f=w1320:u16)
          n641 = Select(t=w1313, s=w1310, f=u16 0) -> (s? t:f=w1308:u16)
          n642 = Select(t=w1311, s=w1310, f=w1314) -> (s? t:f=w1307:u16)
          n643 = Select(t=w1299, s=w1290, f=u16 0) -> (s? t:f=w1293:u16)
          n644 = Select(t=w1297, s=w1290, f=w1300) -> (s? t:f=w1291:u16)
          n645 = Replace Array Subset(array=w1319, new element #1=w1321, index #1=w1304, new element #2=w1320, index #2=w1316, new element #3=w1308, index #3=w1302, new element #4=w1307, index #4=w1309, new element #5=w1293, index #5=w1289, new element #6=w1291, index #6=w1292) -> (w1318:u16[])
        }
        frame 29 {
          # "Audio_L"
          # "Tcycle"
          # "count"
          n646 = call "BRig_dataMTrig_Audio_c_L.vi"() -> ("output_Audio_c_L"=w1329:i32)  [unwired: 11 in]
          n647 = call "BRig_dataMTrig_Audio_T_L.vi"() -> ("output_Audio_T_L"=w1335:i32)  [unwired: 11 in]
          n648 = call "BRig_dataMTrig_CueLed_c.vi"() -> ("output_CueLed_c"=w1350:i32)  [unwired: 11 in]
          n649 = call "BRig_dataMTrig_CueLed_T.vi"() -> ("output_CueLed_T"=w1349:i32)  [unwired: 11 in]
          n650 = call "BRig_dataMTrig_Laser_c_l1.vi"() -> ("output_Laser_c_l1"=w1348:i32)  [unwired: 11 in]
          n651 = call "BRig_dataMTrig_Laser_T_l1.vi"() -> ("output_Laser_T_l1"=w1347:i32)  [unwired: 11 in]
          n652 = call "BRig_dataMTrig_Laser_c_l2.vi"() -> ("output_Laser_c_l2"=w1328:i32)  [unwired: 11 in]
          n653 = call "BRig_dataMTrig_Laser_T_l2.vi"() -> ("output_Laser_T_l2"=w1327:i32)  [unwired: 11 in]
          n654 = Index Array(array=w1367, index #1=w1329, index #2=w1335, index #3=w1350, index #4=w1349, index #5=w1348, index #6=w1347, index #7=w1328, index #8=w1327) -> (element #1=w1333:u16, element #2=w1334:u16, element #3=w1371:u16, element #4=w1370:u16, element #5=w1352:u16, element #6=w1351:u16, element #7=w1342:u16, element #8=w1341:u16)
          n655 = Add(x=w1340, y=w1333) -> (x+y=w1376:u16)
          n656 = Add(x=w1340, y=w1371) -> (x+y=w1373:u16)
          n657 = Add(x=w1340, y=w1352) -> (x+y=w1359:u16)
          n658 = Add(x=w1340, y=w1342) -> (x+y=w1345:u16)
          n659 = Less?(x=w1376, y=w1334) -> (x < y?=w1365:bool)
          n660 = Less?(x=w1373, y=w1370) -> (x < y?=w1364:bool)
          n661 = Less?(x=w1359, y=w1351) -> (x < y?=w1356:bool)
          n662 = Less?(x=w1345, y=w1341) -> (x < y?=w1336:bool)
          n663 = Decrement(x=w1363) -> (x-1=w1377:u16)
          n664 = Decrement(x=w1361) -> (x-1=w1374:u16)
          n665 = Decrement(x=w1357) -> (x-1=w1360:u16)
          n666 = Decrement(x=w1343) -> (x-1=w1346:u16)
          n667 = Select(t=w1376, s=w1365, f=u16 0) -> (s? t:f=w1330:u16)
          n668 = Select(t=w1363, s=w1365, f=w1377) -> (s? t:f=w1332:u16)
          n669 = Select(t=w1373, s=w1364, f=u16 0) -> (s? t:f=w1369:u16)
          n670 = Select(t=w1361, s=w1364, f=w1374) -> (s? t:f=w1368:u16)
          n671 = Select(t=w1359, s=w1356, f=u16 0) -> (s? t:f=w1354:u16)
          n672 = Select(t=w1357, s=w1356, f=w1360) -> (s? t:f=w1353:u16)
          n673 = Select(t=w1345, s=w1336, f=u16 0) -> (s? t:f=w1339:u16)
          n674 = Select(t=w1343, s=w1336, f=w1346) -> (s? t:f=w1337:u16)
          n675 = Replace Array Subset(array=w1367, new element #1=w1330, index #1=w1329, new element #2=w1332, index #2=w1331, new element #3=w1369, index #3=w1350, new element #4=w1368, index #4=w1362, new element #5=w1354, index #5=w1348, new element #6=w1353, index #6=w1355, new element #7=w1339, index #7=w1328, new element #8=w1337, index #8=w1338) -> (w1366:u16[])
        }
        frame 30 {
          # "Audio_R"
          # "Tcycle"
          # "count"
          n676 = call "BRig_dataMTrig_Laser_c_l2.vi"() -> ("output_Laser_c_l2"=w1379:i32)  [unwired: 11 in]
          n677 = call "BRig_dataMTrig_Laser_T_l2.vi"() -> ("output_Laser_T_l2"=w1378:i32)  [unwired: 11 in]
          n678 = call "BRig_dataMTrig_Audio_c_R.vi"() -> ("output_Audio_c_R"=w1422:i32)  [unwired: 11 in]
          n679 = call "BRig_dataMTrig_Audio_T_R.vi"() -> ("output_Audio_T_R"=w1423:i32)  [unwired: 11 in]
          n680 = call "BRig_dataMTrig_CueLed_c.vi"() -> ("output_CueLed_c"=w1394:i32)  [unwired: 11 in]
          n681 = call "BRig_dataMTrig_CueLed_T.vi"() -> ("output_CueLed_T"=w1393:i32)  [unwired: 11 in]
          n682 = call "BRig_dataMTrig_Laser_c_l1.vi"() -> ("output_Laser_c_l1"=w1392:i32)  [unwired: 11 in]
          n683 = call "BRig_dataMTrig_Laser_T_l1.vi"() -> ("output_Laser_T_l1"=w1391:i32)  [unwired: 11 in]
          n684 = Index Array(array=w1412, index #1=w1422, index #2=w1423, index #3=w1394, index #4=w1393, index #5=w1392, index #6=w1391, index #7=w1379, index #8=w1378) -> (element #1=w1425:u16, element #2=w1424:u16, element #3=w1416:u16, element #4=w1415:u16, element #5=w1396:u16, element #6=w1395:u16, element #7=w1386:u16, element #8=w1385:u16)
          n685 = Add(x=w1384, y=w1425) -> (x+y=w1427:u16)
          n686 = Add(x=w1384, y=w1416) -> (x+y=w1418:u16)
          n687 = Add(x=w1384, y=w1396) -> (x+y=w1403:u16)
          n688 = Add(x=w1384, y=w1386) -> (x+y=w1389:u16)
          n689 = Less?(x=w1427, y=w1424) -> (x < y?=w1410:bool)
          n690 = Less?(x=w1418, y=w1415) -> (x < y?=w1409:bool)
          n691 = Less?(x=w1403, y=w1395) -> (x < y?=w1400:bool)
          n692 = Less?(x=w1389, y=w1385) -> (x < y?=w1380:bool)
          n693 = Decrement(x=w1407) -> (x-1=w1428:u16)
          n694 = Decrement(x=w1405) -> (x-1=w1419:u16)
          n695 = Decrement(x=w1401) -> (x-1=w1404:u16)
          n696 = Decrement(x=w1387) -> (x-1=w1390:u16)
          n697 = Select(t=w1427, s=w1410, f=u16 0) -> (s? t:f=w1421:u16)
          n698 = Select(t=w1407, s=w1410, f=w1428) -> (s? t:f=w1420:u16)
          n699 = Select(t=w1418, s=w1409, f=u16 0) -> (s? t:f=w1414:u16)
          n700 = Select(t=w1405, s=w1409, f=w1419) -> (s? t:f=w1413:u16)
          n701 = Select(t=w1403, s=w1400, f=u16 0) -> (s? t:f=w1398:u16)
          n702 = Select(t=w1401, s=w1400, f=w1404) -> (s? t:f=w1397:u16)
          n703 = Select(t=w1389, s=w1380, f=u16 0) -> (s? t:f=w1383:u16)
          n704 = Select(t=w1387, s=w1380, f=w1390) -> (s? t:f=w1381:u16)
          n705 = Replace Array Subset(array=w1412, new element #1=w1421, index #1=w1422, new element #2=w1420, index #2=w1408, new element #3=w1414, index #3=w1394, new element #4=w1413, index #4=w1406, new element #5=w1398, index #5=w1392, new element #6=w1397, index #6=w1399, new element #7=w1383, index #7=w1379, new element #8=w1381, index #8=w1382) -> (w1411:u16[])
        }
        frame 31 {
          # "Audio_R"
          # "Tcycle"
          # "count"
          # "Audio_L"
          # "Tcycle"
          # "count"
          n706 = call "BRig_dataMTrig_Audio_c_L.vi"() -> ("output_Audio_c_L"=w1483:i32)  [unwired: 11 in]
          n707 = call "BRig_dataMTrig_Audio_T_L.vi"() -> ("output_Audio_T_L"=w1488:i32)  [unwired: 11 in]
          n708 = call "BRig_dataMTrig_Audio_c_R.vi"() -> ("output_Audio_c_R"=w1476:i32)  [unwired: 11 in]
          n709 = call "BRig_dataMTrig_Audio_T_R.vi"() -> ("output_Audio_T_R"=w1477:i32)  [unwired: 11 in]
          n710 = call "BRig_dataMTrig_CueLed_c.vi"() -> ("output_CueLed_c"=w1445:i32)  [unwired: 11 in]
          n711 = call "BRig_dataMTrig_CueLed_T.vi"() -> ("output_CueLed_T"=w1444:i32)  [unwired: 11 in]
          n712 = call "BRig_dataMTrig_Laser_c_l2.vi"() -> ("output_Laser_c_l2"=w1430:i32)  [unwired: 11 in]
          n713 = call "BRig_dataMTrig_Laser_T_l2.vi"() -> ("output_Laser_T_l2"=w1429:i32)  [unwired: 11 in]
          n714 = call "BRig_dataMTrig_Laser_c_l1.vi"() -> ("output_Laser_c_l1"=w1443:i32)  [unwired: 11 in]
          n715 = call "BRig_dataMTrig_Laser_T_l1.vi"() -> ("output_Laser_T_l1"=w1442:i32)  [unwired: 11 in]
          n716 = Index Array(array=w1466, index #1=w1483, index #2=w1488, index #3=w1476, index #4=w1477, index #5=w1445, index #6=w1444, index #7=w1443, index #8=w1442, index #9=w1430, index #10=w1429) -> (element #1=w1487:u16, element #2=w1486:u16, element #3=w1479:u16, element #4=w1478:u16, element #5=w1470:u16, element #6=w1469:u16, element #7=w1447:u16, element #8=w1446:u16, element #9=w1437:u16, element #10=w1436:u16)
          n717 = Add(x=w1435, y=w1487) -> (x+y=w1490:u16)
          n718 = Add(x=w1435, y=w1479) -> (x+y=w1481:u16)
          n719 = Add(x=w1435, y=w1470) -> (x+y=w1472:u16)
          n720 = Add(x=w1435, y=w1447) -> (x+y=w1454:u16)
          n721 = Add(x=w1435, y=w1437) -> (x+y=w1440:u16)
          n722 = Less?(x=w1490, y=w1486) -> (x < y?=w1464:bool)
          n723 = Less?(x=w1481, y=w1478) -> (x < y?=w1463:bool)
          n724 = Less?(x=w1472, y=w1469) -> (x < y?=w1462:bool)
          n725 = Less?(x=w1454, y=w1446) -> (x < y?=w1451:bool)
          n726 = Less?(x=w1440, y=w1436) -> (x < y?=w1431:bool)
          n727 = Decrement(x=w1460) -> (x-1=w1491:u16)
          n728 = Decrement(x=w1458) -> (x-1=w1482:u16)
          n729 = Decrement(x=w1456) -> (x-1=w1473:u16)
          n730 = Decrement(x=w1452) -> (x-1=w1455:u16)
          n731 = Decrement(x=w1438) -> (x-1=w1441:u16)
          n732 = Select(t=w1490, s=w1464, f=u16 0) -> (s? t:f=w1485:u16)
          n733 = Select(t=w1460, s=w1464, f=w1491) -> (s? t:f=w1484:u16)
          n734 = Select(t=w1481, s=w1463, f=u16 0) -> (s? t:f=w1475:u16)
          n735 = Select(t=w1458, s=w1463, f=w1482) -> (s? t:f=w1474:u16)
          n736 = Select(t=w1472, s=w1462, f=u16 0) -> (s? t:f=w1468:u16)
          n737 = Select(t=w1456, s=w1462, f=w1473) -> (s? t:f=w1467:u16)
          n738 = Select(t=w1454, s=w1451, f=u16 0) -> (s? t:f=w1449:u16)
          n739 = Select(t=w1452, s=w1451, f=w1455) -> (s? t:f=w1448:u16)
          n740 = Select(t=w1440, s=w1431, f=u16 0) -> (s? t:f=w1434:u16)
          n741 = Select(t=w1438, s=w1431, f=w1441) -> (s? t:f=w1432:u16)
          n742 = Replace Array Subset(array=w1466, new element #1=w1485, index #1=w1483, new element #2=w1484, index #2=w1461, new element #3=w1475, index #3=w1476, new element #4=w1474, index #4=w1459, new element #5=w1468, index #5=w1445, new element #6=w1467, index #6=w1457, new element #7=w1449, index #7=w1443, new element #8=w1448, index #8=w1450, new element #9=w1434, index #9=w1430, new element #10=w1432, index #10=w1433) -> (w1465:u16[])
        }
      }
      "output_Audio_L" <- w59
      "output_Audio_R" <- w58
      "output_CueLed" <- w57
      "output_Laser_l1" <- w56
      "output_Laser_l2" <- w55
      n743 = Replace Array Subset(array=w20, new element #1=w15, index #1=w18, new element #2=w16, index #2=w17) -> (w19:u16[])
      n744 = case shown="3" w49 {
        tunnel: w19 -> [w270 w291 w324 w373]
        tunnel: [w270 w290 w323 w372] -> w54
        tunnel: w53 -> [_ w272 w310 w342]
        tunnel: w48 -> [_ w285 _ w367]
        tunnel: w26 -> [_ w286 _ w368]
        tunnel: w47 -> [_ _ w315 w347]
        tunnel: w21 -> [_ _ w318 w350]
        tunnel: [_ w273 _ w355] -> w44
        tunnel: [_ _ w311 w343] -> w43
        frame 0, Default {
        }
        frame 1 {
          # "N"
          # "state"
          # "count"
          n745 = call "BRig_dataMTrig_Solenoid_c_L.vi"() -> ("output_Solenoid_c_L"=w279:i32)  [unwired: 11 in]
          n746 = call "BRig_dataMTrig_Solenoid_T_L.vi"() -> ("output_Solenoid_T_L"=w284:i32)  [unwired: 11 in]
          n747 = call "BRig_dataMTrig_Solenoid_s_L.vi"() -> ("output_Solenoid_s_L"=w277:i32)  [unwired: 11 in]
          n748 = call "BRig_dataMTrig_Solenoid_Td.vi"() -> ("output_Solenoid_Td"=w289:i32)  [unwired: 11 in]
          n749 = Index Array(array=w291, index #1=w289, index #2=w279, index #3=w284, index #4=w277) -> (element #1=w271:u16, element #2=w283:u16, element #3=w282:u16, element #4=w280:u16)
          n750 = Not Equal To 0?(x=w280) -> (x != 0?=w287:bool)
          n751 = Select(t=w271, s=w287, f=w282) -> (s? t:f=w288:u16)
          n752 = Add(x=w283, y=w272) -> (x+y=w281:u16)
          n753 = Less?(x=w281, y=w288) -> (x < y?=w274:bool)
          n754 = case shown="False" w274 {
            tunnel: w287 -> [w295 w300]
            tunnel: [w297 w301] -> w276
            tunnel: w281 -> [_ w303]
            tunnel: [w296 w303] -> w278
            tunnel: w286 -> [w293 w302]
            tunnel: [w292 w302] -> w275
            tunnel: w280 -> [_ w301]
            tunnel: [_ w299] -> w273
            frame False {
              w296 = u16 0
              n755 = Decrement(x=w293) -> (x-1=w294:u16)
              n756 = Select(t=w296, s=w295, f=u16 1) -> (s? t:f=w297:u16)
              n757 = Select(t=w294, s=w295, f=w293) -> (s? t:f=w292:u16)
            }
            frame True {
              n758 = Not(x=w300) -> (.not. x?=w299:bool)
            }
          }
          n759 = Replace Array Subset(array=w291, new element #1=w275, index #1=w285, new element #2=w278, index #2=w279, new element #3=w276, index #3=w277) -> (w290:u16[])
        }
        frame 2 {
          # "N"
          # "state"
          # "count"
          n760 = call "BRig_dataMTrig_Solenoid_c_R.vi"() -> ("output_Solenoid_c_R"=w308:i32)  [unwired: 11 in]
          n761 = call "BRig_dataMTrig_Solenoid_T_R.vi"() -> ("output_Solenoid_T_R"=w307:i32)  [unwired: 11 in]
          n762 = call "BRig_dataMTrig_Solenoid_s_R.vi"() -> ("output_Solenoid_s_R"=w306:i32)  [unwired: 11 in]
          n763 = call "BRig_dataMTrig_Solenoid_Td.vi"() -> ("output_Solenoid_Td"=w305:i32)  [unwired: 11 in]
          n764 = Index Array(array=w324, index #1=w305, index #2=w308, index #3=w307, index #4=w306) -> (element #1=w304:u16, element #2=w309:u16, element #3=w317:u16, element #4=w316:u16)
          n765 = Not Equal To 0?(x=w316) -> (x != 0?=w321:bool)
          n766 = Select(t=w304, s=w321, f=w317) -> (s? t:f=w322:u16)
          n767 = Add(x=w309, y=w310) -> (x+y=w320:u16)
          n768 = Less?(x=w320, y=w322) -> (x < y?=w319:bool)
          n769 = case shown="False" w319 {
            tunnel: w321 -> [w328 w333]
            tunnel: [w330 w334] -> w312
            tunnel: w320 -> [_ w336]
            tunnel: [w329 w336] -> w313
            tunnel: w318 -> [w326 w335]
            tunnel: [w325 w335] -> w314
            tunnel: w316 -> [_ w334]
            tunnel: [_ w332] -> w311
            frame False {
              w329 = u16 0
              n770 = Decrement(x=w326) -> (x-1=w327:u16)
              n771 = Select(t=w329, s=w328, f=u16 1) -> (s? t:f=w330:u16)
              n772 = Select(t=w327, s=w328, f=w326) -> (s? t:f=w325:u16)
            }
            frame True {
              n773 = Not(x=w333) -> (.not. x?=w332:bool)
            }
          }
          n774 = Replace Array Subset(array=w324, new element #1=w314, index #1=w315, new element #2=w313, index #2=w308, new element #3=w312, index #3=w306) -> (w323:u16[])
        }
        frame 3 {
          # "N"
          # "state"
          # "count"
          # "N"
          # "state"
          # "count"
          n775 = call "BRig_dataMTrig_Solenoid_c_L.vi"() -> ("output_Solenoid_c_L"=w361:i32)  [unwired: 11 in]
          n776 = call "BRig_dataMTrig_Solenoid_T_L.vi"() -> ("output_Solenoid_T_L"=w366:i32)  [unwired: 11 in]
          n777 = call "BRig_dataMTrig_Solenoid_s_L.vi"() -> ("output_Solenoid_s_L"=w359:i32)  [unwired: 11 in]
          n778 = call "BRig_dataMTrig_Solenoid_c_R.vi"() -> ("output_Solenoid_c_R"=w339:i32)  [unwired: 11 in]
          n779 = call "BRig_dataMTrig_Solenoid_T_R.vi"() -> ("output_Solenoid_T_R"=w338:i32)  [unwired: 11 in]
          n780 = call "BRig_dataMTrig_Solenoid_s_R.vi"() -> ("output_Solenoid_s_R"=w337:i32)  [unwired: 11 in]
          n781 = call "BRig_dataMTrig_Solenoid_Td.vi"() -> ("output_Solenoid_Td"=w371:i32)  [unwired: 11 in]
          n782 = Index Array(array=w373, index #1=w371, index #2=w361, index #3=w366, index #4=w359, index #5=w339, index #6=w338, index #7=w337) -> (element #1=w340:u16, element #2=w365:u16, element #3=w364:u16, element #4=w362:u16, element #5=w341:u16, element #6=w349:u16, element #7=w348:u16)
          n783 = Not Equal To 0?(x=w362) -> (x != 0?=w369:bool)
          n784 = Not Equal To 0?(x=w348) -> (x != 0?=w353:bool)
          n785 = Select(t=w340, s=w369, f=w364) -> (s? t:f=w370:u16)
          n786 = Select(t=w340, s=w353, f=w349) -> (s? t:f=w354:u16)
          n787 = Add(x=w365, y=w342) -> (x+y=w363:u16)
          n788 = Add(x=w341, y=w342) -> (x+y=w352:u16)
          n789 = Less?(x=w363, y=w370) -> (x < y?=w356:bool)
          n790 = Less?(x=w352, y=w354) -> (x < y?=w351:bool)
          n791 = case shown="False" w356 {
            tunnel: w369 -> [w389 w394]
            tunnel: [w391 w395] -> w358
            tunnel: w363 -> [_ w397]
            tunnel: [w390 w397] -> w360
            tunnel: w368 -> [w387 w396]
            tunnel: [w386 w396] -> w357
            tunnel: w362 -> [_ w395]
            tunnel: [_ w393] -> w355
            frame False {
              w390 = u16 0
              n792 = Decrement(x=w387) -> (x-1=w388:u16)
              n793 = Select(t=w390, s=w389, f=u16 1) -> (s? t:f=w391:u16)
              n794 = Select(t=w388, s=w389, f=w387) -> (s? t:f=w386:u16)
            }
            frame True {
              n795 = Not(x=w394) -> (.not. x?=w393:bool)
            }
          }
          n796 = case shown="False" w351 {
            tunnel: w353 -> [w377 w382]
            tunnel: [w379 w383] -> w344
            tunnel: w352 -> [_ w385]
            tunnel: [w378 w385] -> w345
            tunnel: w350 -> [w375 w384]
            tunnel: [w374 w384] -> w346
            tunnel: w348 -> [_ w383]
            tunnel: [_ w381] -> w343
            frame False {
              w378 = u16 0
              n797 = Decrement(x=w375) -> (x-1=w376:u16)
              n798 = Select(t=w378, s=w377, f=u16 1) -> (s? t:f=w379:u16)
              n799 = Select(t=w376, s=w377, f=w375) -> (s? t:f=w374:u16)
            }
            frame True {
              n800 = Not(x=w382) -> (.not. x?=w381:bool)
            }
          }
          n801 = Replace Array Subset(array=w373, new element #1=w357, index #1=w367, new element #2=w360, index #2=w361, new element #3=w358, index #3=w359, new element #4=w346, index #4=w347, new element #5=w345, index #5=w339, new element #6=w344, index #6=w337) -> (w372:u16[])
        }
      }
      "output_Solenoid_L" <- w44
      "output_Solenoid_R" <- w43
    }
    frame True {
      n802 = call "BRig_dataMTrig_Audio_T_L.vi"() -> ("output_Audio_T_L"=w1510:i32)  [unwired: 11 in]
      n803 = call "BRig_dataMTrig_Audio_T_R.vi"() -> ("output_Audio_T_R"=w1509:i32)  [unwired: 11 in]
      n804 = call "BRig_dataMTrig_CueLed_T.vi"() -> ("output_CueLed_T"=w1508:i32)  [unwired: 11 in]
      n805 = call "BRig_dataMTrig_Laser_T_l1.vi"() -> ("output_Laser_T_l1"=w1507:i32)  [unwired: 11 in]
      n806 = call "BRig_dataMTrig_Laser_T_l2.vi"() -> ("output_Laser_T_l2"=w1506:i32)  [unwired: 11 in]
      n807 = call "BRig_dataMTrig_Solenoid_T_L.vi"() -> ("output_Solenoid_T_L"=w1505:i32)  [unwired: 11 in]
      n808 = call "BRig_dataMTrig_Solenoid_T_R.vi"() -> ("output_Solenoid_T_R"=w1504:i32)  [unwired: 11 in]
      n809 = Index Array(array=w1492, index #1=w1510, index #2=w1509, index #3=w1508, index #4=w1507, index #5=w1506, index #6=w1505, index #7=w1504) -> (element #1=w1499:u16, element #2=w1498:u16, element #3=w1501:u16, element #4=w1495:u16, element #5=w1494:u16, element #6=w1502:u16, element #7=w1503:u16)
      n810 = Not Equal To 0?(x=w1495) -> (x != 0?=w1496:bool)
      n811 = Select(t=w1495, s=w1496, f=w1494) -> (s? t:f=w1493:u16)
      n812 = Not Equal To 0?(x=w1499) -> (x != 0?=w1500:bool)
      n813 = Select(t=w1499, s=w1500, f=w1498) -> (s? t:f=w1497:u16)
      n814 = local write "Audio_T"(w1497) -> ()
      n815 = local write "CueLed_T"(w1501) -> ()
      n816 = local write "Laser_T"(w1493) -> ()
      n817 = local write "Solenoid_T_L"(w1502) -> ()
      n818 = local write "Solenoid_T_R"(w1503) -> ()
    }
  }
  "output_dataMTrig" <- w3
